vi "Certification Authority.vi"() -> ()   [LabVIEW 2013, in "Certification Authority.lvclass"]
uses:
  Certification Authority.lvclass
  certificate -- cluster.ctl
  certificate signature request (CA) -- cluster.ctl
  encryption key -- cluster.ctl
  initca -- cluster.ctl
  certificate signature request (Server) -- cluster.ctl
  <vilib>/Platform/browser.llb/Open URL in Default Browser (string).vi
  <vilib>/Platform/browser.llb/Open URL in Default Browser (path).vi
  <userlib>/_OpenG.lib/file/file.llb/Build Path - Traditional__ogtk.vi
  <userlib>/_OpenG.lib/file/file.llb/File Exists - Scalar__ogtk.vi
  <userlib>/_OpenG.lib/file/file.llb/Convert File Extension (String)__ogtk.vi
panel:
  in  "Tab Control":T1(tab)
  in  "Root Certificate":path
  in  "Root Private Key":path
  in  "Open Certificates Folder":bool
  in  "Open GitHub Project Page":bool
  in  "Hosts":string[](array[string])=["lvtls-ca.example", "www.lvtls-ca.example"]
  in  "Common Name":string="lvtls-ca.example"
  in  "Generate Root Certificate":bool
  out "CFSSL App found":bool
  out "Root Certificate found":bool
  in  "Generate Server Certificates":bool
  in  "Servers":cluster{"hosts":string[], "name":string}[](array[cluster])
  out "Certificates":T2(array[cluster])
  in  "Certificates and Keys":i32(listbox)
  out "Selected Certificate":string
  # "ROOT (CERTIFICATE AUTHORITY)\nIf you have a root certificate and private key, import it to generate server certificate files.\nIf you don't have a root certificate, fill in the fields in section 2 and generate one."
  # "GENERATE ROOT CERTIFICATE\nIf you don't have a root certificate, fill in the fields below and generate one."
  # "3- SERVERS\nList each server you want to create certificates for."
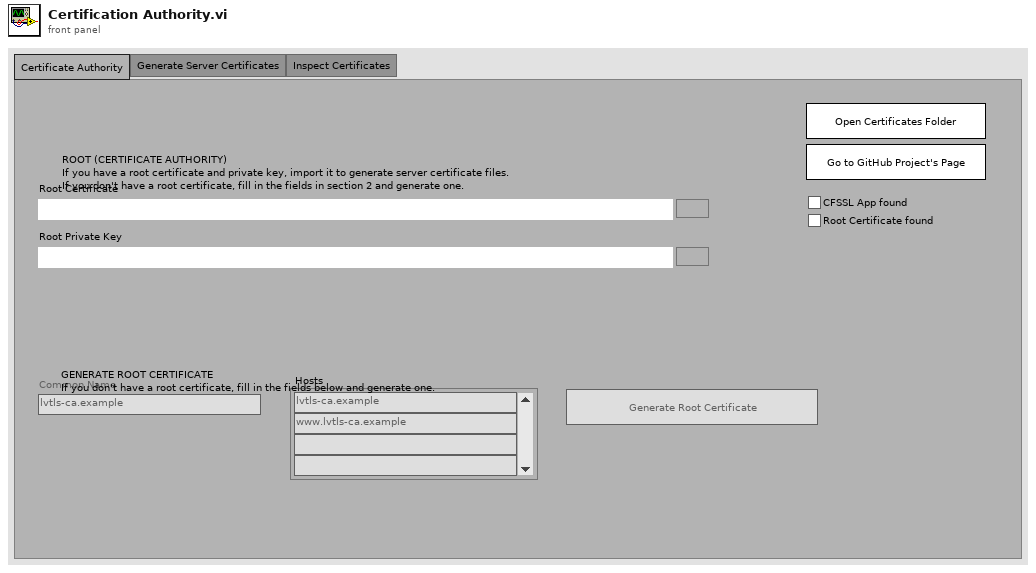
[diagram p1: front panel]
types:
  T1 = enum32{"Certificate Authority", "Generate Server Certificates", "Inspect Certificates"}
  T2 = cluster{"Type":string, "Decoded Certificate":string}[]
  T3 = enum32{"Invalid", "Standard", "Closed", "Hidden", "Minimized", "Maximized"}
  T4 = enum32{"invalid app kind", "Development System", "Run Time System", "Student Edition", "Embedded LabVIEW", "Evaluation", "Custom"}
  T5 = enum16{"open", "replace", "create", "open or create", "replace or create", "replace or create with confirmation"}
  T6 = typedef "Certification Authority.lvclass/certificate signature request (CA) -- cluster.ctl" = cluster{"CN":string, "hosts":string[], "key":T7, "ca":T8}
  T7 = typedef "Certification Authority.lvclass/encryption key -- cluster.ctl" = cluster{"algo":string, "size":u32}
  T8 = typedef "Certification Authority.lvclass/initca -- cluster.ctl" = cluster{"pathlen":u8, "expiry":string}
  T9 = typedef "Certification Authority.lvclass/certificate signature request (Server) -- cluster.ctl" = cluster{"CN":string, "hosts":string[], "key":T7}
  T10 = typedef "Certification Authority.lvclass/certificate -- cluster.ctl" = cluster{"cert":string, "csr":string, "key":string}
  T11 = cluster{"Core":cluster{"Current VI Reference":refnum<vi>, "Close Panel on Exit?":bool}, "CA":T10, "Server":T10, "cfssl path":path, "temp folder":path, "Certificates Folder":path, "Root name":string, "Root Certificate":path, "Root Private Key":path, "Active CN":string, "Active Hosts":string[], "next":i32, "Processing Queue":cluster{"hosts":string[], "name":string}[]}
  T12 = cluster{"Current VI Reference":refnum<vi>, "Close Panel on Exit?":bool}
  T13 = cluster{"Type":string, "Decoded String":string}[]
  T14 = enum8{"Enabled", "Disabled", "Disabled and Grayed Out"}
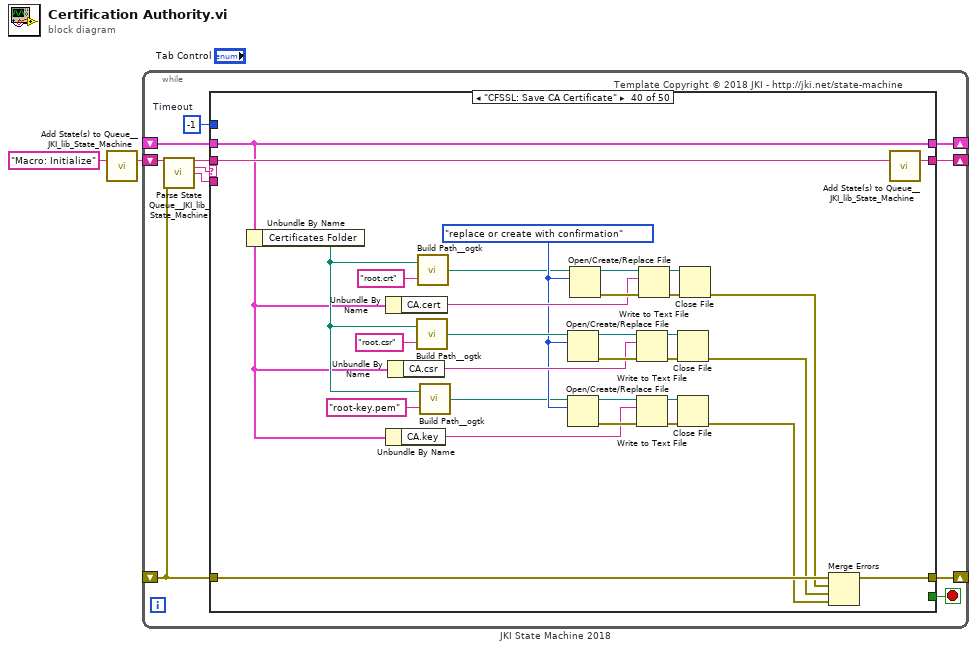
[diagram p0: block diagram]
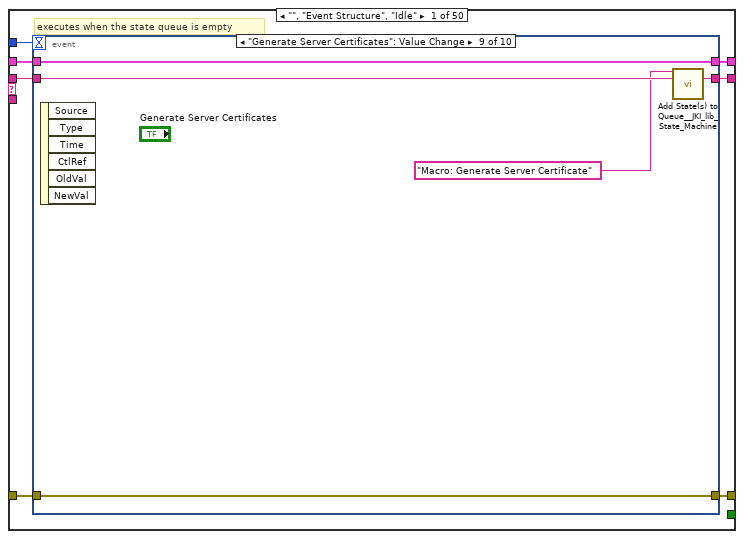
[diagram p2: hidden frame]
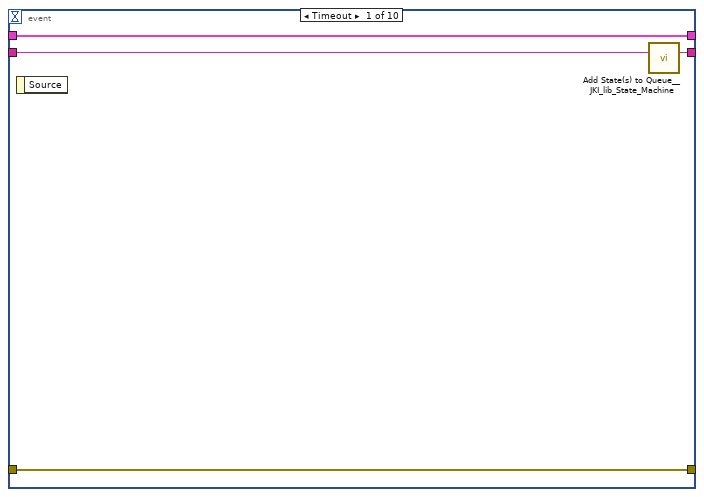
[diagram p3: hidden frame]
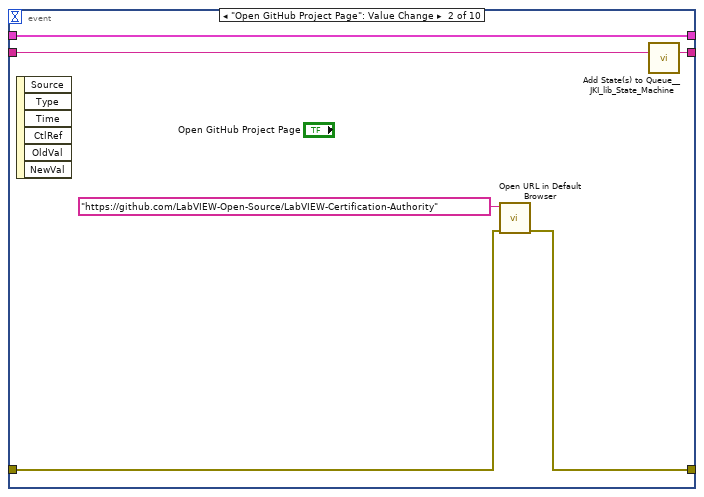
[diagram p4: hidden frame]
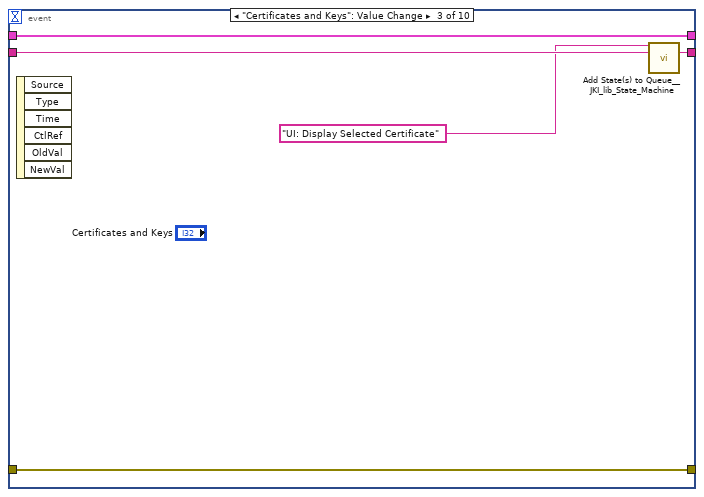
[diagram p5: hidden frame]
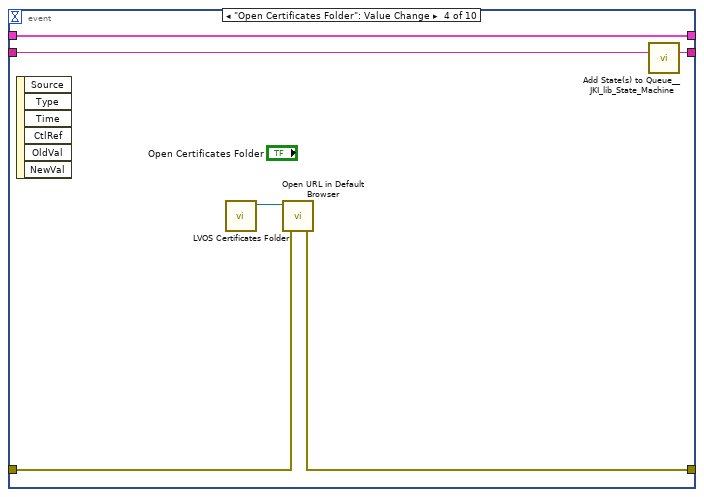
[diagram p6: hidden frame]
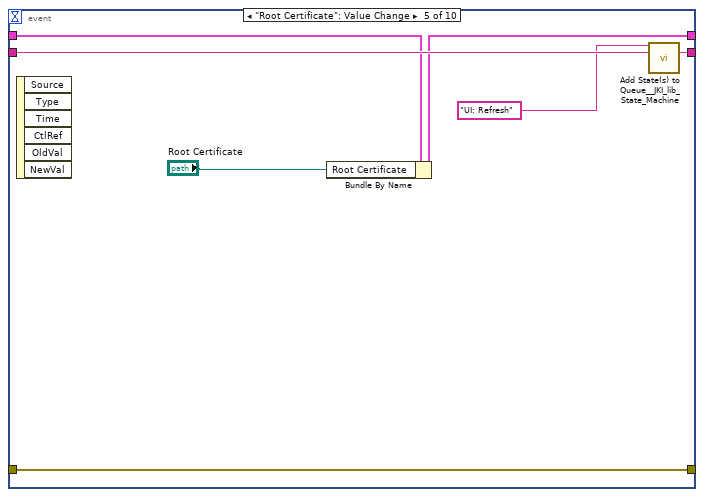
[diagram p7: hidden frame]
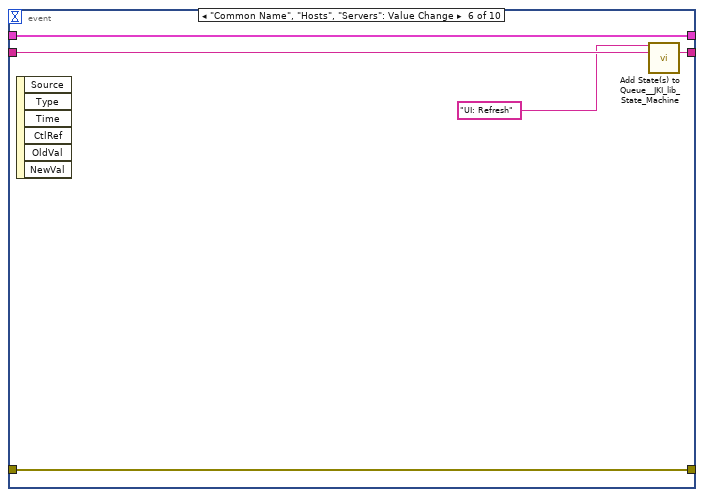
[diagram p8: hidden frame]
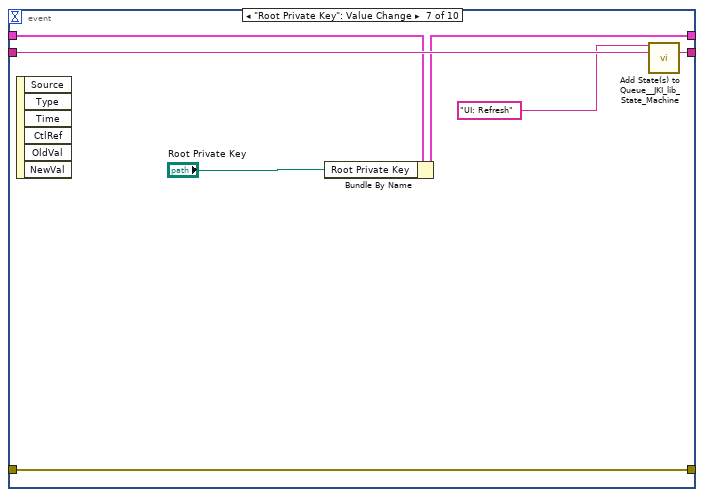
[diagram p9: hidden frame]
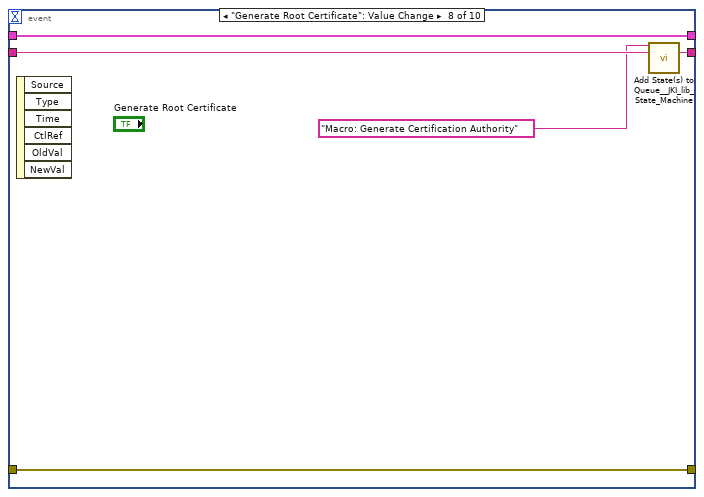
[diagram p10: hidden frame]
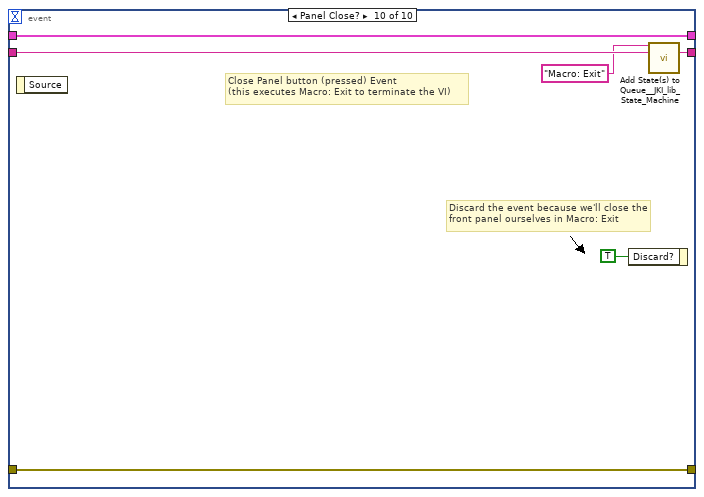
[diagram p11: hidden frame]
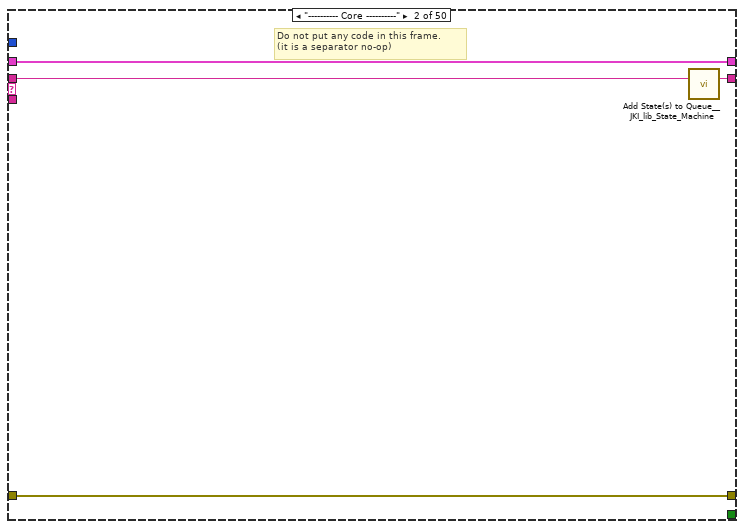
[diagram p12: hidden frame]
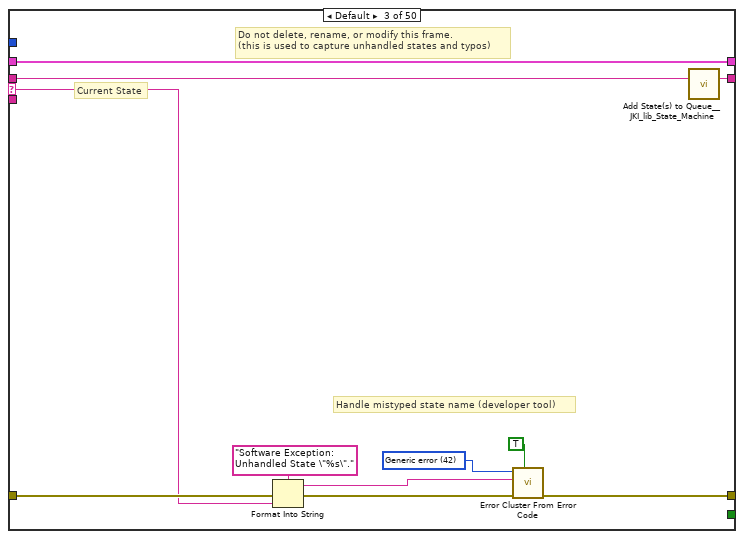
[diagram p13: hidden frame]
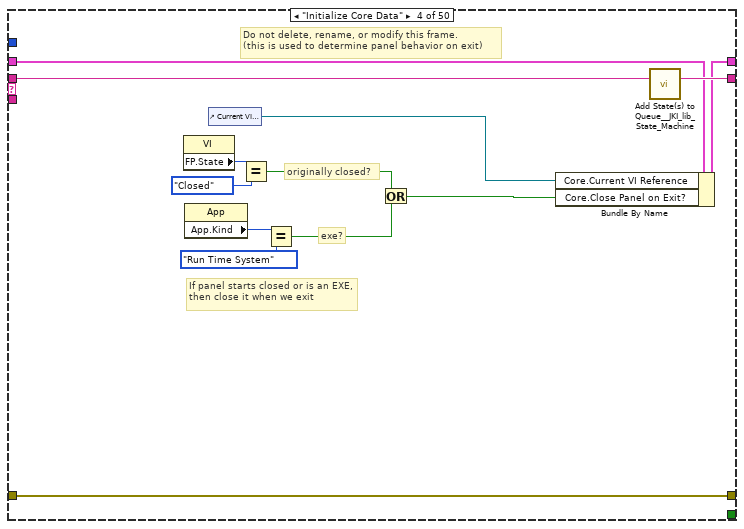
[diagram p14: hidden frame]
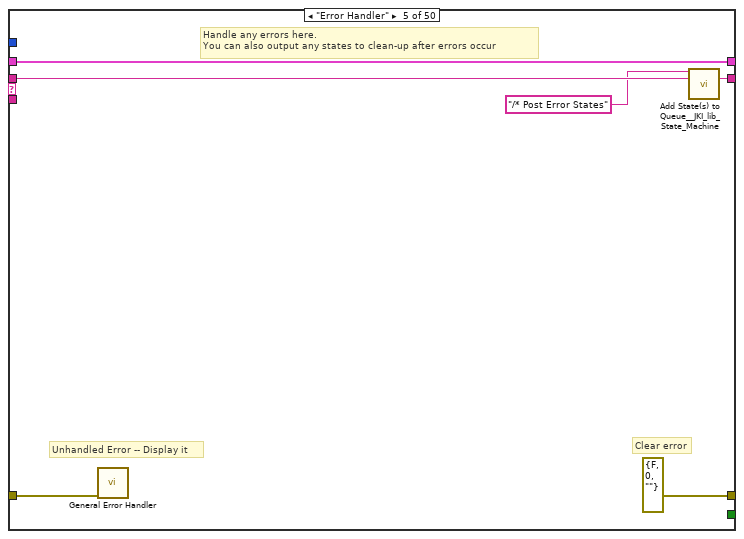
[diagram p15: hidden frame]
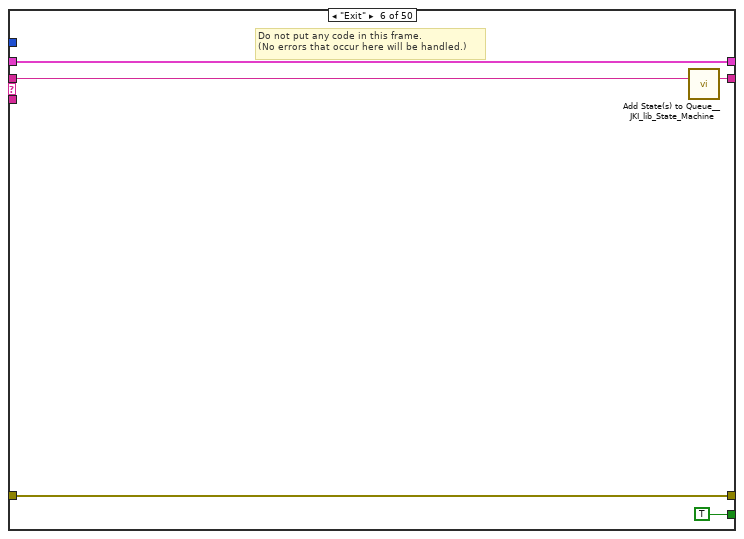
[diagram p16: hidden frame]
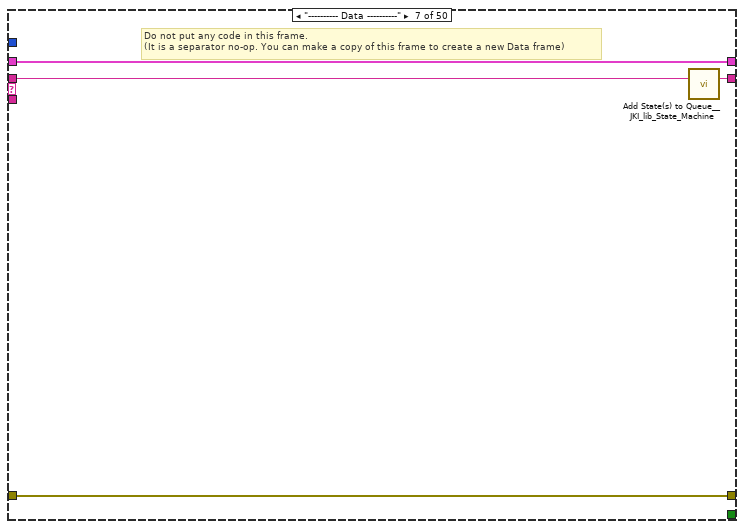
[diagram p17: hidden frame]
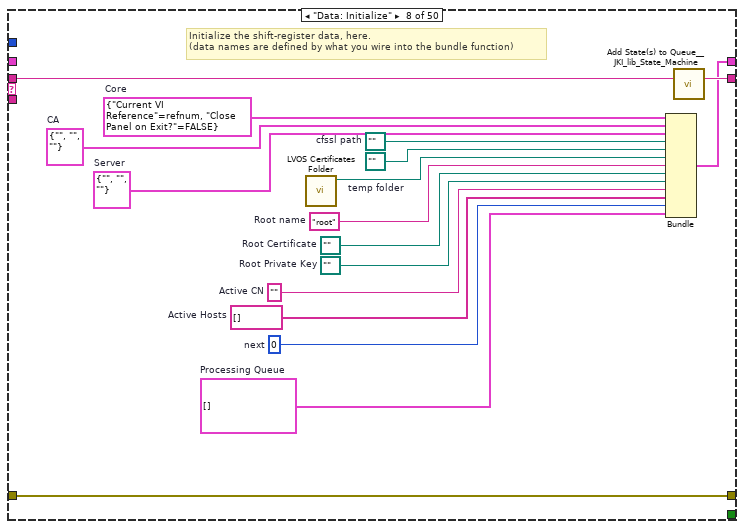
[diagram p18: hidden frame]
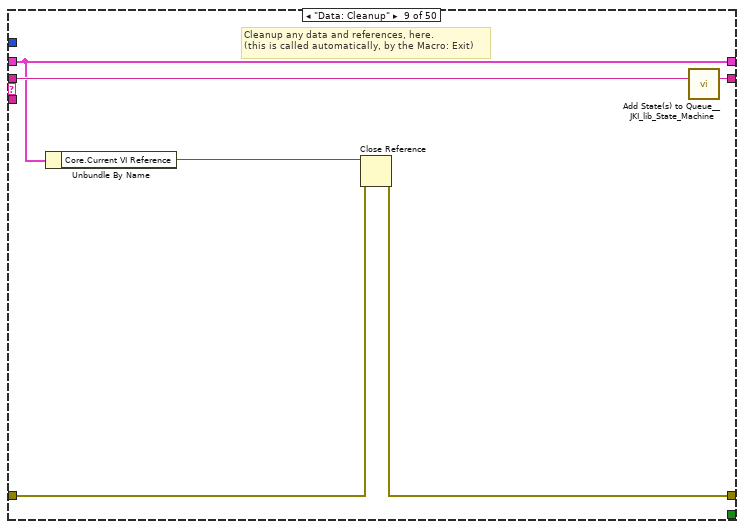
[diagram p19: hidden frame]
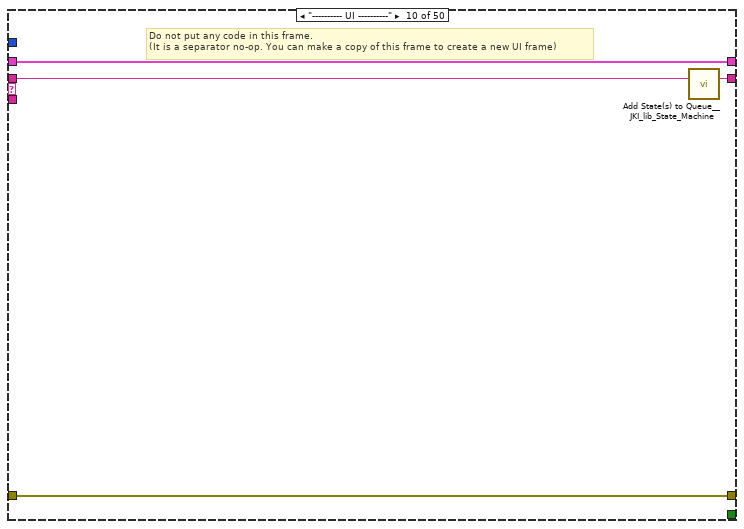
[diagram p20: hidden frame]
diagram:
  n1 = call <vilib>:"Add State(s) to Queue__JKI_lib_State_Machine.vi"("State(s) in (\"\")"="Macro: Initialize") -> ("States Out"=w2:string)  [unwired: 14 in]
  n2 = while "JKI State Machine 2018" {
    shift-right: [w6] -> _
    shift-left: _ -> [w5]
    shift-right: [w9] -> _
    shift-left: _ -> [w3]
    shift-right: [w8] -> _
    shift-left: w2 -> [w10]
    stop <- w7 stop-if-true
    w4 = -1  # Timeout
    # "Template Copyright © 2018 JKI - http://jki.net/state-machine"
    n3 = call <vilib>:"Parse State Queue__JKI_lib_State_Machine.vi"("State Queue"=w10, "Error In (no error)"=w3) -> ("Remaining States"=w12:string, "Current State"=w13:string, "Arguments"=w11:string)  [unwired: 11 in]
    n4 = case shown="\"CFSSL: Save CA Certificate\"" w13 {
      selector: w13 -> [_ _ w81 _ _ _ _ _ _ _ _ _ _ _ _ _ _ _ _ _ _ _ _ _ _ _ _ _ _ _ _ _ _ _ _ _ _ _ _ _ _ _ _ _ _ _ _ _ _ _]
      tunnel: w12 -> [w20 w80 w85 w104 w110 w115 w119 w136 w142 w146 w155 w166 w175 w230 w234 w238 w243 w249 w260 w329 w334 w339 w347 w352 w361 w366 w377 w381 w392 w405 w415 w442 w457 w472 w495 w516 w533 w543 w557 w588 w611 w637 w660 w692 w709 w726 w743 w760 w777 w794]
      tunnel: w11 -> [_ _ _ _ _ _ _ _ _ _ _ _ _ _ _ _ _ w244 w254 _ _ _ _ _ _ _ _ _ _ _ _ _ _ _ _ _ _ _ _ _ _ _ _ _ _ _ _ _ _ _]
      tunnel: w5 -> [w18 w77 w83 w97 w107 w113 w116 _ w137 w143 w153 w164 w173 w200 w231 w235 w240 w247 w256 w326 w331 w336 w343 w349 w358 w363 w374 w378 w389 w403 w413 w438 w446 w462 w493 w514 w526 w538 w555 w558 w604 w633 w650 w675 w701 w718 w735 w752 w769 w786]
      tunnel: [w17 w78 w87 w101 errorcluster {"status"=FALSE, "code"=0, "source"=""} ("error out") w112 w117 w133 w138 w144 w149 w161 w170 w228 w232 w236 w241 w245 w257 w327 w332 w337 w345 w350 w359 w364 w375 w379 w390 w398 w409 w440 w443 w459 w473 w502 w519 w534 w546 w561 w606 w634 w639 w676 w696 w713 w730 w747 w764 w781] -> w9
      tunnel: w3 -> [w16 w78 w86 w101 w106 w112 w117 w133 w139 w144 w150 w162 w170 w228 w232 w236 w241 w246 w258 w327 w332 w337 w345 w350 w359 w364 w375 w379 w390 w399 w408 w440 w444 w460 w474 w503 w520 w534 w544 w565 w607 w635 w642 w679 w698 w715 w732 w749 w766 w783]
      tunnel: [w19 w79 w84 w103 w109 w114 w118 w135 w141 w145 w154 w165 w174 w229 w233 w237 w242 w248 w259 w328 w333 w338 w346 w351 w360 w365 w376 w380 w391 w404 w414 w441 w456 w471 w494 w515 w532 w542 w556 w587 w610 w636 w659 w691 w708 w725 w742 w759 w776 w793] -> w8
      tunnel: [_ _ _ _ _ TRUE _ _ _ _ _ _ _ _ _ _ _ _ _ _ _ _ _ _ _ _ _ _ _ _ _ _ _ _ _ _ _ _ _ _ _ _ _ _ _ _ _ _ _ _] -> w7
      tunnel: [w15 w77 w83 w102 w107 w113 w116 w134 w137 w143 w153 w164 w173 w200 w231 w235 w240 w247 w256 w326 w331 w336 w342 w349 w358 w363 w374 w378 w388 w402 w413 w439 w447 w463 w493 w514 w526 w541 w555 w558 w603 w632 w650 w675 w701 w718 w735 w752 w769 w786] -> w6
      tunnel: w4 -> [w14 _ _ _ _ _ _ _ _ _ _ _ _ _ _ _ _ _ _ _ _ _ _ _ _ _ _ _ _ _ _ _ _ _ _ _ _ _ _ _ _ _ _ _ _ _ _ _ _ _]
      frame "", "Event Structure", "Idle" {
        # "executes when the state queue is empty"
        n5 = event shown="[8] \"Generate Server Certificates\": Value Change" {
          selector: _ -> [_ _ _ _ _ _ _ _ _ _]
          dyn-events: _ -> [_ _ _ _ _ _ _ _ _ _]
          timeout: w14 -> [_ _ _ _ _ _ _ _ _ _]
          tunnel: w20 -> [w24 w30 w35 w41 w48 w53 w60 w65 w70 w76]
          tunnel: [w23 w29 w34 w40 w47 w52 w59 w64 w69 w75] -> w19
          tunnel: w18 -> [w21 w28 w32 w39 w45 w49 w57 w62 w67 w73]
          tunnel: [w22 w25 w33 w36 w46 w51 w58 w63 w68 w74] -> w17
          tunnel: w16 -> [w22 w26 w33 w37 w46 w51 w58 w63 w68 w74]
          tunnel: [w21 w28 w32 w39 w44 w49 w56 w62 w67 w73] -> w15
          event Timeout {
            n6 = event-data() -> ()  [unwired: 1 in, 1 out]
            n7 = call <vilib>:"Add State(s) to Queue__JKI_lib_State_Machine.vi"("State(s) in (\"\")"=w24) -> ("States Out"=w23:string)  [unwired: 14 in]
          }
          event "Open GitHub Project Page": Value Change {
            n8 = event-data() -> ()  [unwired: 1 in, 6 out]
            n9 = call-poly <vilib>:"Open URL in Default Browser.vi"("error in (no error)"=w26, "URL"="https://github.com/LabVIEW-Open-Source/LabVIEW-Certification-Authority") -> ("error out"=w25:errorcluster)  [unwired: 4 in, 1 out]
            n10 = call <vilib>:"Add State(s) to Queue__JKI_lib_State_Machine.vi"("State(s) in (\"\")"=w30) -> ("States Out"=w29:string)  [unwired: 14 in]
          }
          event "Certificates and Keys": Value Change {
            n11 = event-data() -> ()  [unwired: 1 in, 6 out]
            n12 = call <vilib>:"Add State(s) to Queue__JKI_lib_State_Machine.vi"("State(s) in Front (\"\")"="UI: Display Selected Certificate", "State(s) in (\"\")"=w35) -> ("States Out"=w34:string)  [unwired: 13 in]
          }
          event "Open Certificates Folder": Value Change {
            n13 = event-data() -> ()  [unwired: 1 in, 6 out]
            n14 = call "LVOS Certificates Folder.vi"() -> ("Certificates Folder"=w38:path)  [unwired: 10 in, 1 out]
            n15 = call-poly <vilib>:"Open URL in Default Browser.vi"("error in (no error)"=w37, "path"=w38) -> ("error out"=w36:errorcluster)  [unwired: 4 in, 1 out]
            n16 = call <vilib>:"Add State(s) to Queue__JKI_lib_State_Machine.vi"("State(s) in (\"\")"=w41) -> ("States Out"=w40:string)  [unwired: 14 in]
          }
          event "Root Certificate": Value Change {
            n17 = event-data() -> ()  [unwired: 1 in, 6 out]
            n18 = Bundle By Name(cluster=w45, "Root Certificate"="Root Certificate") -> (w44:T11)
            n19 = call <vilib>:"Add State(s) to Queue__JKI_lib_State_Machine.vi"("State(s) in Front (\"\")"="UI: Refresh", "State(s) in (\"\")"=w48) -> ("States Out"=w47:string)  [unwired: 13 in]
          }
          event "Common Name", "Hosts", "Servers": Value Change {
            n20 = event-data() -> ()  [unwired: 1 in, 6 out]
            n21 = call <vilib>:"Add State(s) to Queue__JKI_lib_State_Machine.vi"("State(s) in Front (\"\")"="UI: Refresh", "State(s) in (\"\")"=w53) -> ("States Out"=w52:string)  [unwired: 13 in]
          }
          event "Root Private Key": Value Change {
            n22 = event-data() -> ()  [unwired: 1 in, 6 out]
            n23 = Bundle By Name(cluster=w57, "Root Private Key"="Root Private Key") -> (w56:T11)
            n24 = call <vilib>:"Add State(s) to Queue__JKI_lib_State_Machine.vi"("State(s) in Front (\"\")"="UI: Refresh", "State(s) in (\"\")"=w60) -> ("States Out"=w59:string)  [unwired: 13 in]
          }
          event "Generate Root Certificate": Value Change {
            n25 = event-data() -> ()  [unwired: 1 in, 6 out]
            n26 = call <vilib>:"Add State(s) to Queue__JKI_lib_State_Machine.vi"("State(s) in Front (\"\")"="Macro: Generate Certification Authority", "State(s) in (\"\")"=w65) -> ("States Out"=w64:string)  [unwired: 13 in]
          }
          event "Generate Server Certificates": Value Change {
            n27 = event-data() -> ()  [unwired: 1 in, 6 out]
            n28 = call <vilib>:"Add State(s) to Queue__JKI_lib_State_Machine.vi"("State(s) in Front (\"\")"="Macro: Generate Server Certificate", "State(s) in (\"\")"=w70) -> ("States Out"=w69:string)  [unwired: 13 in]
          }
          event Panel Close? {
            # "Discard the event because we'll close the front panel ourselves in Macro: Exit"
            # "Close Panel button (pressed) Event\n(this executes Macro: Exit to terminate the VI)"
            n29 = event-data() -> ()  [unwired: 1 in, 1 out]
            n30 = event-data("Discard?"=TRUE) -> ()  [unwired: 1 in, 1 out]
            n31 = call <vilib>:"Add State(s) to Queue__JKI_lib_State_Machine.vi"("State(s) in Front (\"\")"="Macro: Exit", "State(s) in (\"\")"=w76) -> ("States Out"=w75:string)  [unwired: 13 in]
          }
        }
      }
      frame "---------- Core ----------" {
        # "Do not put any code in this frame.\n(it is a separator no-op)"
        n32 = call <vilib>:"Add State(s) to Queue__JKI_lib_State_Machine.vi"("State(s) in (\"\")"=w80) -> ("States Out"=w79:string)  [unwired: 14 in]
      }
      frame Default {
        w90 = 42 items=["No error", "Argument error", "Memory is full", "Out of zone", "End of file", "File already open", "Generic file I/O error", "File not found", "File permission error", "Disk is full", "Duplicate path", "Too many files open", "System feature not enabled", "Resource file not found", "Cannot add resource", "Resource not found", "Image not found", "Image memory error", "Pen does not exist", "Config type invalid", "Config token not found", "Config parse error", "Config memory error", "Bad external code format", "Bad external code offset", "External code not present", "Null window", "Destroy window error", "Null menu", "Print aborted", "Bad print record", "Print driver error", "Windows error during printing", "Memory error during printing", "Print dialog error", "Generic print error", "Invalid device refnum", "Device not found", "Device parameter error", "Device unit error", "Cannot open device", "Device call aborted", "Generic error", "Cancelled by user", "Object ID too low", "Object ID too high", "Object not in heap", "Unknown heap", "Unknown object (invalid DefProc)", "Unknown object (DefProc not in table)", "Message out of range", "Invalid (null) method", "Unknown message", "Manager call not supported", "Bad address", "Network operation in progress", "Network operation timed out", "Connection is busy", "Network attribute not supported", "Network error", "Address in use", "System out of memory", "Connection aborted", "Connection refused", "Not connected", "Already connected", "Connection closed", "Initialization error (interapplication manager)", "Bad occurrence", "Wait on unbound occurrence handler", "Occurrence queue overflow", "Datalog type conflict", "Unused", "Unrecognized type (interapplication manager)", "Memory corrupt", "Failed to make temporary DLL", "Old CIN version", "Drag socket not found", "Failed to load drop-object", "Failed to register OLE object", "Failed to release OLE object", "Format specifier type mismatch", "Unknown format specifier", "Too few format specifiers", "Too many format specifiers", "Scan failed", "Newer CIN version", "Error converting to variant", "Runtime menu error", "Password tampered", "Variant attribute not found", "Incompatible variant data type", "Event data is not available", "Event Store is not present", "Occurrence is not found", "Event Queue is not created", "Event info is not available", "Refnum passed is NULL", "Error retrieving Class GUID", "Error retrieving CoClass GUID", "Error retrieving TypeLib GUID.", "Bad built application magic bytes.", "Specific driver is different from the specific driver associated with the Logical Name.", "There is no session opened to the class driver.", "Max Error", "MAX - Error with config objects", "MAX - Error loading configuration", "MAX - Group not supported"]
        # "Current State"
        # "Do not delete, rename, or modify this frame.\n(this is used to capture unhandled states and typos)"
        # "Handle mistyped state name (developer tool)"
        n33 = Format Into String(format string="Software Exception: Unhandled State \"%s\"." ("message"), error in=w86, w81) -> (resulting string=w89:string, error out=w88:errorcluster)  [unwired: 1 in]
        n34 = call <vilib>:"Error Cluster From Error Code.vi"("show call chain? (False)"=TRUE, "error in (no error)"=w88, "error message (\"\")"=w89, "error code (0)"=w90) -> ("error out"=w87:errorcluster)  [unwired: 5 in]
        n35 = call <vilib>:"Add State(s) to Queue__JKI_lib_State_Machine.vi"("State(s) in (\"\")"=w85) -> ("States Out"=w84:string)  [unwired: 14 in]
      }
      frame "Initialize Core Data" {
        # "Do not delete, rename, or modify this frame.\n(this is used to determine panel behavior on exit)"
        # "originally closed?"
        # "exe?"
        # "If panel starts closed or is an EXE, then close it when we exit"
        n36 = property class="VI"() -> ("FP.State"=w94:T3)  [unwired: 2 in, 2 out]
        n37 = property class="App"() -> ("App.Kind"=w100:T4)  [unwired: 2 in, 2 out]
        n38 = control-ref of="Current VI Reference"() -> (w95:refnum<vi>)
        n39 = Equal?(x=w94, y=T3."Closed" ("Front Panel Window:State")) -> (x = y?=w92:bool)
        n40 = Equal?(x=w100, y=T4."Run Time System" ("Application:Kind")) -> (x = y?=w98:bool)
        n41 = Or(x=w92, y=w98) -> (x .or. y?=w96:bool)
        n42 = Bundle By Name(cluster=w97, "Core.Current VI Reference"=w95, "Core.Close Panel on Exit?"=w96) -> (w102:T11)
        n43 = call <vilib>:"Add State(s) to Queue__JKI_lib_State_Machine.vi"("State(s) in (\"\")"=w104) -> ("States Out"=w103:string)  [unwired: 14 in]
      }
      frame "Error Handler" {
        # "Unhandled Error -- Display it"
        # "Handle any errors here.\nYou can also output any states to clean-up after errors occur"
        # "Clear error"
        n44 = call <vilib>:"General Error Handler.vi"("error in (no error)"=w106) -> ()  [unwired: 10 in, 5 out]
        n45 = call <vilib>:"Add State(s) to Queue__JKI_lib_State_Machine.vi"("State(s) in Front (\"\")"="/* Post Error States", "State(s) in (\"\")"=w110) -> ("States Out"=w109:string)  [unwired: 13 in]
      }
      frame "Exit" {
        # "Do not put any code in this frame.\n(No errors that occur here will be handled.)"
        n46 = call <vilib>:"Add State(s) to Queue__JKI_lib_State_Machine.vi"("State(s) in (\"\")"=w115) -> ("States Out"=w114:string)  [unwired: 14 in]
      }
      frame "---------- Data ----------" {
        # "Do not put any code in this frame.\n(It is a separator no-op. You can make a copy of this frame to create a new Data frame)"
        n47 = call <vilib>:"Add State(s) to Queue__JKI_lib_State_Machine.vi"("State(s) in (\"\")"=w119) -> ("States Out"=w118:string)  [unwired: 14 in]
      }
      frame "Data: Initialize" {
        w120 = cluster{"hosts":string[], "name":string}[] []  # Processing Queue
        w121 = 0  # next
        w123 = string[] []  # Active Hosts
        w124 = ""  # Active CN
        w125 = path ""  # Root Private Key
        w126 = path ""  # Root Certificate
        w127 = "root"  # Root name
        w128 = path ""  # temp folder
        w129 = path ""  # cfssl path
        w130 = T10 {"cert"="", "csr"="", "key"=""}  # Server
        w131 = T10 {"cert"="", "csr"="", "key"=""}  # CA
        w132 = T12 {"Current VI Reference"=refnum, "Close Panel on Exit?"=FALSE}  # Core
        # "Initialize the shift-register data, here.\n(data names are defined by what you wire into the bundle function)"
        n48 = call "LVOS Certificates Folder.vi"() -> ("Certificates Folder"=w122:path)  [unwired: 10 in, 1 out]
        n49 = Bundle("Core"=w132, "CA"=w131, "Server"=w130, "cfssl path"=w129, "temp folder"=w128, "Certificates Folder"=w122, "Root name"=w127, "Root Certificate"=w126, "Root Private Key"=w125, "Active CN"=w124, "Active Hosts"=w123, "next"=w121, "Processing Queue"=w120) -> (w134:T11)  [unwired: 1 in]
        n50 = call <vilib>:"Add State(s) to Queue__JKI_lib_State_Machine.vi"("State(s) in (\"\")"=w136) -> ("States Out"=w135:string)  [unwired: 14 in]
      }
      frame "Data: Cleanup" {
        # "Cleanup any data and references, here.\n(this is called automatically, by the Macro: Exit)"
        n51 = Unbundle By Name(w137) -> ("Core.Current VI Reference"=w140:refnum<vi>)
        n52 = Close Reference(reference=w140, error in (no error)=w139) -> (error out=w138:errorcluster)
        n53 = call <vilib>:"Add State(s) to Queue__JKI_lib_State_Machine.vi"("State(s) in (\"\")"=w142) -> ("States Out"=w141:string)  [unwired: 14 in]
      }
      frame "---------- UI ----------" {
        # "Do not put any code in this frame.\n(It is a separator no-op. You can make a copy of this frame to create a new UI frame)"
        n54 = call <vilib>:"Add State(s) to Queue__JKI_lib_State_Machine.vi"("State(s) in (\"\")"=w146) -> ("States Out"=w145:string)  [unwired: 14 in]
      }
      frame "UI: Initialize" {
        # "Initialize the User Interface, here.\n(this is called automatically, by the Macro: Init)"
        n55 = property on="Certificates and Keys" class="LstBox (strict)"("Item Names"=string[] []) -> ()  [unwired: 2 in, 2 out]
        n56 = local write "Tab Control"(0) -> ()
        n57 = call "LVOS Certificates Folder.vi"() -> ("Certificates Folder"=w152:path)  [unwired: 10 in, 1 out]
        n58 = call <userlib>:"Create Dir if Non-Existant__ogtk.vi"("error in (no error)"=w150, "Directory Path"=w152) -> ("error out"=w149:errorcluster, "dup Directory Path"=w151:path)  [unwired: 7 in, 1 out]
        n59 = invoke on="Servers" class="Arr (strict)" method="Reinit To Default"() -> ()  [unwired: 3 in, 3 out]
        n60 = property on="Root Private Key" class="Path"("StartPath"=w151) -> ()  [unwired: 2 in, 2 out]
        n61 = property on="Root Certificate" class="Path"("StartPath"=w151) -> ()  [unwired: 2 in, 2 out]
        n62 = call <vilib>:"Add State(s) to Queue__JKI_lib_State_Machine.vi"("State(s) in (\"\")"=w155) -> ("States Out"=w154:string)  [unwired: 14 in]
      }
      frame "UI: List Certificates" {
        n63 = call "LVOS Certificates Folder.vi"() -> ("Certificates Folder"=w163:path)  [unwired: 10 in, 1 out]
        n64 = call <userlib>:"Create Dir if Non-Existant__ogtk.vi"("error in (no error)"=w162, "Directory Path"=w163) -> ("error out"=w161:errorcluster, "dup Directory Path"=w160:path)  [unwired: 7 in, 1 out]
        n65 = call <userlib>:"List Directory__ogtk.vi"("pattern"="*.pem; *.crt; *.csr", "directory path"=w160) -> ("file names"=w158:string[])  [unwired: 2 in, 3 out]
        n66 = Sort 1D Array(array=w158) -> (sorted array=w157:string[])
        n67 = property on="Certificates and Keys" class="LstBox (strict)"("Item Names"=w157, "Value"=-1 ("Trusted Certificates")) -> ()  [unwired: 2 in, 2 out]
        n68 = call <vilib>:"Add State(s) to Queue__JKI_lib_State_Machine.vi"("State(s) in (\"\")"=w166) -> ("States Out"=w165:string)  [unwired: 14 in]
      }
      frame "UI: Display Selected Certificate" {
        n69 = property on="Certificates and Keys" class="LstBox (strict)"() -> ("Item Names"=w172:string[], "Value"=w171:i32)  [unwired: 2 in, 2 out]
        n70 = Index Array(array=w172, index=w171) -> (element=w169:string)
        n71 = case shown="Default" w169 {
          selector: w169 -> [w182 _]
          tunnel: [w176 _] -> w168
          frame Default {
            n72 = call "LVOS Certificates Folder.vi"() -> ("Certificates Folder"=w183:path)  [unwired: 10 in, 1 out]
            n73 = call-poly <userlib>:"Build Path__ogtk.vi"("name or relative path"=w182, "base path"=w183) -> ("appended path"=w178:path)
            n74 = call-poly <userlib>:"File Exists__ogtk.vi"("file path"=w178) -> ("is directory"=w181:bool, "exists"=w180:bool)  [unwired: 6 in]
            n75 = Empty String/Path?(string/path=w178) -> (empty?=w179:bool)
            n76 = Compound Arithmetic op=AND(invert w181, w180, invert w179) -> (w177:bool)
            n77 = case shown="True" w177 {
              tunnel: w178 -> [_ w185]
              tunnel: [_ w184] -> w176
              frame False {
              }
              frame True {
                n78 = Open/Create/Replace File(file path (use dialog)=w185, operation (0:open)=T5."open", access (0:read/write)=enum16{"read/write", "read-only", "write-only"}."read-only") -> (refnum out=w190:refnum<file>, error out=w191:errorcluster)  [unwired: 3 in, 1 out]
                n79 = Read from Text File(file (use dialog)=w190, error in=w191) -> (refnum out=w188:refnum<file>, text=w184:string, error out=w189:errorcluster)  [unwired: 2 in, 1 out]
                n80 = Close File(refnum=w188, error in=w189) -> ()  [unwired: 2 out]
              }
            }
          }
          frame "" {
          }
        }
        "Selected Certificate" <- w168
        n81 = call "Inspect Certificate.vi"("Certificate string"=w168) -> ("Certificates"=→"Certificates":T13)  [unwired: 10 in]
        n82 = call <vilib>:"Add State(s) to Queue__JKI_lib_State_Machine.vi"("State(s) in (\"\")"=w175) -> ("States Out"=w174:string)  [unwired: 14 in]
      }
      frame "UI: Refresh" {
        w205 = T14."Disabled and Grayed Out" ("Disabled")
        w204 = T14."Enabled" ("Disabled")
        n83 = Unbundle By Name(w200) -> ("Certificates Folder"=w225:path)
        n84 = Unbundle By Name(w200) -> ("Root Certificate"=w202:path, "Root Private Key"=w201:path)
        n85 = local read "Common Name"() -> (w209:string)
        n86 = local read "Servers"() -> (w222:cluster{"hosts":string[], "name":string}[])
        n87 = Unbundle By Name(w200) -> ("cfssl path"=w199:path)
        n88 = local read "Hosts"() -> (w208:string[])
        n89 = Not A Number/Path/Refnum?(number/path/refnum=w199) -> (NaN/Path/Refnum?=w194:bool)
        n90 = local write "Root Private Key"(w201) -> ()
        n91 = call-poly <userlib>:"File Exists__ogtk.vi"("file path"=w225) -> ("is directory"=w223:bool, "exists"=w224:bool)  [unwired: 6 in]
        n92 = Empty String/Path?(string/path=w225) -> (empty?=w226:bool)
        n93 = Empty Array?(array=w222) -> (empty?=w227:bool)
        n94 = Empty String/Path?(string/path=w209) -> (empty?=w207:bool)
        n95 = local write "Root Certificate"(w202) -> ()
        n96 = call-poly <userlib>:"File Exists__ogtk.vi"("file path"=w202) -> ("is directory"=w219:bool, "exists"=w218:bool)  [unwired: 6 in]
        n97 = call-poly <userlib>:"File Exists__ogtk.vi"("file path"=w201) -> ("is directory"=w214:bool, "exists"=w215:bool)  [unwired: 6 in]
        n98 = Empty String/Path?(string/path=w202) -> (empty?=w217:bool)
        n99 = Empty String/Path?(string/path=w201) -> (empty?=w216:bool)
        n100 = Empty Array?(array=w208) -> (empty?=w206:bool)
        n101 = Compound Arithmetic op=AND(invert w219, w218, invert w217) -> (w213:bool)
        n102 = Compound Arithmetic op=AND(invert w214, w215, invert w216) -> (w212:bool)
        n103 = Compound Arithmetic op=AND(w213, w212) -> (w192:bool)
        "Root Certificate found" <- w192
        n104 = Not(x=w194) -> (.not. x?=→"CFSSL App found":bool)
        n105 = Not(x=w192) -> (.not. x?=w196:bool)
        n106 = Compound Arithmetic op=AND(w196, invert w194) -> (w197:bool)
        n107 = Compound Arithmetic op=AND(w192, w223, w224, invert w226, invert w227, invert w194) -> (w220:bool)
        n108 = Compound Arithmetic op=AND(w196, invert w194) -> (w195:bool)
        n109 = Compound Arithmetic op=AND(invert w207, invert w206, w196, invert w194) -> (w198:bool)
        n110 = Select(t=w204, s=w195, f=w205) -> (s? t:f=w210:T14)
        n111 = Select(t=w204, s=w197, f=w205) -> (s? t:f=w211:T14)
        n112 = Select(t=w204, s=w198, f=w205) -> (s? t:f=w203:T14)
        n113 = Select(t=w204, s=w220, f=w205) -> (s? t:f=w221:T14)
        n114 = property on="Generate Root Certificate" class="Bool"("DisabledEnum"=w203) -> ()  [unwired: 2 in, 2 out]
        n115 = property on="Generate Server Certificates" class="Bool"("DisabledEnum"=w221) -> ()  [unwired: 2 in, 2 out]
        n116 = property on="Common Name" class="Str"("DisabledEnum"=w210) -> ()  [unwired: 2 in, 2 out]
        n117 = property on="hostname" class="Str"("DisabledEnum"=w211) -> ()  [unwired: 2 in, 2 out]
        n118 = call <vilib>:"Add State(s) to Queue__JKI_lib_State_Machine.vi"("State(s) in (\"\")"=w230) -> ("States Out"=w229:string)  [unwired: 14 in]
      }
      frame "UI: Display CA" {
        n119 = Unbundle By Name(w231) -> ()  [unwired: 1 out]
        n120 = call <vilib>:"Add State(s) to Queue__JKI_lib_State_Machine.vi"("State(s) in (\"\")"=w234) -> ("States Out"=w233:string)  [unwired: 14 in]
      }
      frame "UI: Display Server Cert" {
        n121 = Unbundle By Name(w235) -> ()  [unwired: 1 out]
        n122 = call <vilib>:"Add State(s) to Queue__JKI_lib_State_Machine.vi"("State(s) in (\"\")"=w238) -> ("States Out"=w237:string)  [unwired: 14 in]
      }
      frame "UI: Show Temporary Folder" {
        n123 = Unbundle By Name(w240) -> ("temp folder"=w239:path)
        n124 = call-poly <vilib>:"Open URL in Default Browser.vi"("path"=w239) -> ()  [unwired: 5 in, 2 out]
        n125 = call <vilib>:"Add State(s) to Queue__JKI_lib_State_Machine.vi"("State(s) in (\"\")"=w243) -> ("States Out"=w242:string)  [unwired: 14 in]
      }
      frame "UI: Cursor Set" {
        # "Argument"
        # "Set and Unset Cursor Busy.\n(Usage: \"UI: Cursor Set >> Busy|Idle\")"
        n126 = case shown="\"Idle\", Default" w244 {
          tunnel: w246 -> [w251 w253]
          tunnel: [w250 w252] -> w245
          frame "Idle", Default {
            n127 = call <vilib>:"Unset Busy.vi"("error in (no error)"=w251) -> ("error out"=w250:errorcluster)  [unwired: 10 in]
          }
          frame "Busy" {
            n128 = call <vilib>:"Set Busy.vi"("error in (no error)"=w253) -> ("error out"=w252:errorcluster)  [unwired: 9 in, 1 out]
          }
        }
        n129 = call <vilib>:"Add State(s) to Queue__JKI_lib_State_Machine.vi"("State(s) in (\"\")"=w249) -> ("States Out"=w248:string)  [unwired: 14 in]
      }
      frame "UI: Front Panel State" {
        # "Argument"
        # "Set Front Panel Open or Closed\n(Usage: \"UI: Front Panel State >> Open|Close\")"
        n130 = Unbundle By Name(w256) -> ("Core.Current VI Reference"=w255:refnum<vi>)
        n131 = case shown="\"Minimize\", \"Minimized\"" w254 {
          tunnel: w258 -> [w266 w281 w292 w305 w318]
          tunnel: [w268 w282 w294 w307 w320] -> w257
          tunnel: w255 -> [w267 w279 w293 w306 w319]
          frame "Open", "Standard", Default {
            w261 = T3."Standard" ("State")
            n132 = property class="VI"(reference=w267, error in=w266) -> (reference out=w264:refnum<vi>, error out=w265:errorcluster, "FP.State"=w263:T3)
            n133 = Not Equal?(x=w263, y=w261) -> (x != y?=w262:bool)
            n134 = case shown="True" w262 {
              tunnel: [w272 w274] -> w268
              tunnel: w265 -> [w271 w274]
              tunnel: w264 -> [w270 _]
              tunnel: w261 -> [w269 _]
              frame True {
                n135 = invoke class="VI" method="FP.Open"(reference=w270, error in=w271, "Activate"=TRUE, "State"=w269) -> (error out=w272:errorcluster)  [unwired: 1 in, 4 out]
              }
              frame False {
              }
            }
          }
          frame "Close", "Closed" {
            n136 = property class="VI"(reference=w279, error in=w281) -> (reference out=w278:refnum<vi>, error out=w280:errorcluster, "FP.State"=w276:T3)
            n137 = Not Equal?(x=w276, y=T3."Closed" ("Front Panel Window:State")) -> (x != y?=w275:bool)
            n138 = case shown="True" w275 {
              tunnel: [w283 w286] -> w282
              tunnel: w280 -> [w283 w285]
              tunnel: w278 -> [_ w284]
              frame False {
              }
              frame True {
                n139 = invoke class="VI" method="FP.Close"(reference=w284, error in=w285) -> (error out=w286:errorcluster)  [unwired: 1 in, 2 out]
              }
            }
          }
          frame "Hidden", "Hide" {
            w287 = T3."Hidden" ("State")
            n140 = property class="VI"(reference=w293, error in=w292) -> (reference out=w290:refnum<vi>, error out=w291:errorcluster, "FP.State"=w289:T3)
            n141 = Not Equal?(x=w289, y=w287) -> (x != y?=w288:bool)
            n142 = case shown="True" w288 {
              tunnel: [w298 w299] -> w294
              tunnel: w291 -> [w297 w299]
              tunnel: w290 -> [w296 _]
              tunnel: w287 -> [w295 _]
              frame True {
                n143 = invoke class="VI" method="FP.Open"(reference=w296, error in=w297, "State"=w295) -> (error out=w298:errorcluster)  [unwired: 2 in, 4 out]
              }
              frame False {
              }
            }
          }
          frame "Minimize", "Minimized" {
            w300 = T3."Minimized" ("State")
            n144 = property class="VI"(reference=w306, error in=w305) -> (reference out=w303:refnum<vi>, error out=w304:errorcluster, "FP.State"=w302:T3)
            n145 = Not Equal?(x=w302, y=w300) -> (x != y?=w301:bool)
            n146 = case shown="True" w301 {
              tunnel: [w311 w312] -> w307
              tunnel: w304 -> [w310 w312]
              tunnel: w303 -> [w309 _]
              tunnel: w300 -> [w308 _]
              frame True {
                n147 = invoke class="VI" method="FP.Open"(reference=w309, error in=w310, "State"=w308) -> (error out=w311:errorcluster)  [unwired: 2 in, 4 out]
              }
              frame False {
              }
            }
          }
          frame "Maximize", "Maximized" {
            w313 = T3."Maximized" ("State")
            n148 = property class="VI"(reference=w319, error in=w318) -> (reference out=w316:refnum<vi>, error out=w317:errorcluster, "FP.State"=w315:T3)
            n149 = Not Equal?(x=w315, y=w313) -> (x != y?=w314:bool)
            n150 = case shown="True" w314 {
              tunnel: [w324 w325] -> w320
              tunnel: w317 -> [w323 w325]
              tunnel: w316 -> [w322 _]
              tunnel: w313 -> [w321 _]
              frame True {
                n151 = invoke class="VI" method="FP.Open"(reference=w322, error in=w323, "State"=w321) -> (error out=w324:errorcluster)  [unwired: 2 in, 4 out]
              }
              frame False {
              }
            }
          }
        }
        n152 = call <vilib>:"Add State(s) to Queue__JKI_lib_State_Machine.vi"("State(s) in (\"\")"=w260) -> ("States Out"=w259:string)  [unwired: 14 in]
      }
      frame "---------- Macro ----------" {
        # "Do not put any code in this frame.\n(It is a separator no-op. You can make a copy of this frame to create a new Macro frame)"
        n153 = call <vilib>:"Add State(s) to Queue__JKI_lib_State_Machine.vi"("State(s) in (\"\")"=w329) -> ("States Out"=w328:string)  [unwired: 14 in]
      }
      frame "Macro: Initialize" {
        w330 = "Data: Initialize\nInitialize Core Data\nUI: Initialize\nUI: Front Panel State >> Open\n\nCFSSL: Find EXE\nCFSSL: Load Certification Authority\nCFSSL: Read CA Certificates\nCFSSL: Validate CA Certificates\nCFSSL: Create Temp Folder\nUI: List Certificates\nUI: Display Selected Certificate\nUI: Refresh"  # Data: Initialize Initialize Core Data UI: Initialize UI: Front Panel State >> Open  CFSSL: Find EXE CFSSL: Load Certification Authority CFSSL: Read CA Certificates CFSSL: Validate CA Certificates CFSSL: Create Temp Folder UI: List Certificates UI: Display Selected Certificate UI: Refresh
        # "Initialization Macro\n(This is called once, when the VI starts)"
        n154 = call <vilib>:"Add State(s) to Queue__JKI_lib_State_Machine.vi"("State(s) in Front (\"\")"=w330, "State(s) in (\"\")"=w334) -> ("States Out"=w333:string)  [unwired: 13 in]
      }
      frame "Macro: Generate Certification Authority" {
        n155 = call <vilib>:"Add State(s) to Queue__JKI_lib_State_Machine.vi"("State(s) in Front (\"\")"="CFSSL: Create Temp Folder\nCFSSL: Prepare CA Request File\nCFSSL: Generate Certification Authority\nCFSSL: Save CA Certificate\nCFSSL: Load Certification Authority\nCFSSL: Read CA Certificates\nCFSSL: Validate CA Certificates\nUI: Refresh\nUI: List Certificates\nUI: Display Selected Certificate", "State(s) in (\"\")"=w339) -> ("States Out"=w338:string)  [unwired: 13 in]
      }
      frame "Macro: Generate Server Certificate" {
        n156 = Bundle By Name(cluster=w343, "Processing Queue"="Servers") -> (w342:T11)
        n157 = call <vilib>:"Add State(s) to Queue__JKI_lib_State_Machine.vi"("State(s) in Front (\"\")"="CFSSL: Create Temp Folder\nCFSSL: Prepare Gencert Config File\nCFSSL: Copy Temporary CA Certificate\n\nMacro: Process Next Server", "State(s) in (\"\")"=w347, "State(s) at Back (\"\")"="UI: Refresh\nUI: List Certificates\nUI: Display Selected Certificate") -> ("States Out"=w346:string)  [unwired: 12 in]
      }
      frame "Macro: Export Root Bundle" {
        n158 = call <vilib>:"Add State(s) to Queue__JKI_lib_State_Machine.vi"("State(s) in Front (\"\")"="CFSSL: Export Root Certificate\nCFSSL: Export Root Private Key\nCFSSL: Export Root Signing Request", "State(s) in (\"\")"=w352) -> ("States Out"=w351:string)  [unwired: 13 in]
      }
      frame "Macro: Process Next Server" {
        n159 = Unbundle By Name(w358) -> ("Processing Queue"=w357:cluster{"hosts":string[], "name":string}[])
        n160 = Empty Array?(array=w357) -> (empty?=w356:bool)
        n161 = Select(t="UI: Refresh", s=w356, f="CFSSL: Load Next Server\nCFSSL: Prepare Server Request File\nCFSSL: Generate Server Certificate\nCFSSL: Save Temporary Server Certificate\nMacro: Process Next Server") -> (s? t:f=w353:string)
        n162 = call <vilib>:"Add State(s) to Queue__JKI_lib_State_Machine.vi"("State(s) in Front (\"\")"=w353, "State(s) in (\"\")"=w361) -> ("States Out"=w360:string)  [unwired: 13 in]
      }
      frame "Macro: Export Server Bundle" {
        n163 = call <vilib>:"Add State(s) to Queue__JKI_lib_State_Machine.vi"("State(s) in Front (\"\")"="CFSSL: Export Server Certificate\nCFSSL: Export Server Private Key\nCFSSL: Export Server Signing Request", "State(s) in (\"\")"=w366) -> ("States Out"=w365:string)  [unwired: 13 in]
      }
      frame "Macro: Exit" {
        # "Exit Macro\n(This is called once, when the VI exits)"
        n164 = Unbundle By Name(w374) -> ("Core.Close Panel on Exit?"=w373:bool)
        n165 = Select(t="UI: Front Panel State >> Close", s=w373, f="") -> (s? t:f=w370:string)
        n166 = call <vilib>:"Add State(s) to Queue__JKI_lib_State_Machine.vi"("State(s) in Front (\"\")"="CFSSL: Delete Temp Folder", "State(s) in (\"\")"=w370, "State(s) at Back (\"\")"="Data: Cleanup\nExit") -> ("States Out"=w368:string)  [unwired: 12 in]
        n167 = call <vilib>:"Add State(s) to Queue__JKI_lib_State_Machine.vi"("State(s) in Front (\"\")"=w368, "State(s) in (\"\")"=w377) -> ("States Out"=w376:string)  [unwired: 13 in]
      }
      frame "---------- Cloudflare SSL ----------" {
        n168 = call <vilib>:"Add State(s) to Queue__JKI_lib_State_Machine.vi"("State(s) in (\"\")"=w381) -> ("States Out"=w380:string)  [unwired: 14 in]
      }
      frame "CFSSL: Find EXE" {
        # "Linux\nMac\nnull\nPharLap\nVxWorks\nWin"
        n169 = disable-structure shown="OS==Win" {
          disable-tunnel: [w393 _] -> w383
          frame condition #0 (active) {
            n170 = call "LVOS Certificates Folder.vi"() -> ("cfssl path"=w395:path)  [unwired: 10 in, 1 out]
            n171 = call <userlib>:"Create Dir if Non-Existant__ogtk.vi"("Directory Path"=w395) -> ("dup Directory Path"=w396:path)  [unwired: 8 in, 2 out]
            n172 = Build Path(base path=w396, name or relative path=path "cfssl.exe") -> (appended path=w393:path)
          }
          frame condition #1 {
          }
        }
        n173 = call-poly <userlib>:"File Exists__ogtk.vi"("file path"=w383) -> ("is directory"=w387:bool, "exists"=w386:bool)  [unwired: 6 in]
        n174 = Compound Arithmetic op=OR(invert w387, w386) -> (w385:bool)
        n175 = Select(t=w383, s=w385, f=path "") -> (s? t:f=w384:path)
        n176 = Bundle By Name(cluster=w389, "cfssl path"=w384) -> (w388:T11)
        n177 = call <vilib>:"Add State(s) to Queue__JKI_lib_State_Machine.vi"("State(s) in (\"\")"=w392) -> ("States Out"=w391:string)  [unwired: 14 in]
      }
      frame "CFSSL: Create Temp Folder" {
        n178 = call <userlib>:"Temporary Directory__ogtk.vi"("Relative path (.)"=path "LV_CFSSL") -> ("Temporary Directory (+ Relative)"=w400:path)
        n179 = call <userlib>:"Create Dir if Non-Existant__ogtk.vi"("error in (no error)"=w399, "Directory Path"=w400) -> ("error out"=w398:errorcluster, "dup Directory Path"=w397:path)  [unwired: 7 in, 1 out]
        n180 = Bundle By Name(cluster=w403, "temp folder"=w397) -> (w402:T11)
        n181 = call <vilib>:"Add State(s) to Queue__JKI_lib_State_Machine.vi"("State(s) in (\"\")"=w405) -> ("States Out"=w404:string)  [unwired: 14 in]
      }
      frame "CFSSL: Delete Temp Folder" {
        n182 = Unbundle By Name(w413) -> ("temp folder"=w407:path)
        n183 = Empty String/Path?(string/path=w407) -> (empty?=w406:bool)
        n184 = call-poly <userlib>:"File Exists__ogtk.vi"("file path"=w407) -> ("is directory"=w411:bool, "exists"=w412:bool)  [unwired: 6 in]
        n185 = Compound Arithmetic op=AND(w411, w412, invert w406) -> (w410:bool)
        n186 = case shown="True" w410 {
          tunnel: w407 -> [_ w420]
          tunnel: [w416 w418] -> w409
          tunnel: w408 -> [w416 w419]
          frame False {
          }
          frame True {
            w417 = TRUE ("Recursive? (FALSE)")
            n187 = call <userlib>:"Delete Recursive__ogtk.vi"("error in (no error)"=w419, "Ignore Read-Only? (FALSE)"=w417, "Recursive? (FALSE)"=w417, "Path"=w420) -> ("error out"=w418:errorcluster)  [unwired: 6 in, 1 out]
          }
        }
        n188 = call <vilib>:"Add State(s) to Queue__JKI_lib_State_Machine.vi"("State(s) in (\"\")"=w415) -> ("States Out"=w414:string)  [unwired: 14 in]
      }
      frame "CFSSL: Load Certification Authority" {
        n189 = Unbundle By Name(w438) -> ("Certificates Folder"=w422:path)
        n190 = Build Path(base path=w422, name or relative path="root.crt") -> (appended path=w423:path)
        n191 = Build Path(base path=w422, name or relative path="root-key.pem") -> (appended path=w421:path)
        n192 = call-poly <userlib>:"File Exists__ogtk.vi"("file path"=w423) -> ("is directory"=w436:bool, "exists"=w435:bool)  [unwired: 6 in]
        n193 = Empty String/Path?(string/path=w423) -> (empty?=w434:bool)
        n194 = call-poly <userlib>:"File Exists__ogtk.vi"("file path"=w421) -> ("is directory"=w426:bool, "exists"=w427:bool)  [unwired: 6 in]
        n195 = Empty String/Path?(string/path=w421) -> (empty?=w428:bool)
        n196 = Compound Arithmetic op=AND(invert w436, w435, invert w434) -> (w433:bool)
        n197 = Compound Arithmetic op=AND(invert w426, w427, invert w428) -> (w429:bool)
        n198 = Select(t=w423, s=w433, f=path "") -> (s? t:f=w431:path)
        n199 = Select(t=w421, s=w429, f=path "") -> (s? t:f=w424:path)
        n200 = Bundle By Name(cluster=w438, "Root Certificate"=w431, "Root Private Key"=w424) -> (w439:T11)
        n201 = call <vilib>:"Add State(s) to Queue__JKI_lib_State_Machine.vi"("State(s) in (\"\")"=w442) -> ("States Out"=w441:string)  [unwired: 14 in]
      }
      frame "CFSSL: Generate Certification Authority" {
        n202 = Unbundle By Name(w446) -> ("cfssl path"=w452:path, "temp folder"=w451:path)
        n203 = Format Into String(format string="\"%s\" gencert -initca csr-ca.json", w452) -> (resulting string=w454:string)  [unwired: 2 in, 1 out]
        n204 = call <vilib>:"System Exec.vi"("run minimized? (F)"=TRUE, "error in (no error)"=w444, "working directory"=w451, "command line"=w454) -> ("error out"=w449:errorcluster, "standard output"=w450:string)  [unwired: 4 in, 2 out]
        n205 = Unbundle By Name(w446) -> ("CA"=w445:T10)
        n206 = Unflatten From JSON(JSON string=w450, type and defaults=w445, error in (no error)=w449) -> (value=w448:T10, error out=w443:errorcluster)  [unwired: 4 in]
        n207 = Bundle By Name(cluster=w446, "CA"=w448) -> (w447:T11)
        n208 = call <vilib>:"Add State(s) to Queue__JKI_lib_State_Machine.vi"("State(s) in (\"\")"=w457) -> ("States Out"=w456:string)  [unwired: 14 in]
      }
      frame "CFSSL: Generate Server Certificate" {
        n209 = Unbundle By Name(w462) -> ("cfssl path"=w468:path, "temp folder"=w467:path)
        n210 = Format Into String(format string="\"%s\" gencert -ca ca.pem -ca-key ca-key.pem -config config.json csr-server.json" ("command line"), w468) -> (resulting string=w469:string)  [unwired: 2 in, 1 out]
        n211 = call <vilib>:"System Exec.vi"("run minimized? (F)"=TRUE, "error in (no error)"=w460, "working directory"=w467, "command line"=w469) -> ("error out"=w465:errorcluster, "standard output"=w466:string)  [unwired: 4 in, 2 out]
        n212 = Unbundle By Name(w462) -> ("Server"=w461:T10)
        n213 = Unflatten From JSON(JSON string=w466, type and defaults=w461, error in (no error)=w465) -> (value=w464:T10, error out=w459:errorcluster)  [unwired: 4 in]
        n214 = Bundle By Name(cluster=w462, "Server"=w464) -> (w463:T11)
        n215 = call <vilib>:"Add State(s) to Queue__JKI_lib_State_Machine.vi"("State(s) in (\"\")"=w472) -> ("States Out"=w471:string)  [unwired: 14 in]
      }
      frame "CFSSL: Prepare CA Request File" {
        (unwired) "{\n    \"CN\": \"lvtls-ca.example\",\n    \"hosts\": [\"lvtls-ca.example\"],\n    \"key\": {\"algo\": \"ecdsa\", \"size\": 256},\n    \"names\": [],\n    \"ca\": {\"pathlen\": 1, \"expiry\": \"143800h\"}\n}" ("name or relative path")
        # "https://github.com/cloudflare/cfssl/wiki/Creating-a-new-CSR"
        n216 = Unbundle By Name(w493) -> ("temp folder"=w492:path)
        n217 = call-poly <userlib>:"Build Path__ogtk.vi"("name or relative path"="csr-ca.json", "base path"=w492) -> ("appended path"=w481:path)
        n218 = Bundle By Name(cluster=T6 {"CN"="", "hosts"=[], "key"={"algo"="ecdsa", "size"=256}, "ca"={"pathlen"=0, "expiry"=""}} ("CSR"), "CN"="Common Name", "hosts"="Hosts", "key.algo"="ecdsa", "key.size"=u32 256, "ca.pathlen"=u8 1, "ca.expiry"="143800h") -> (w487:T6)
        n219 = Flatten To JSON(anything=w487, error in (no error)=w474) -> (JSON string=w479:string, 11:w475:errorcluster)  [unwired: 1 in]
        n220 = Open/Create/Replace File(file path (use dialog)=w481, error in=w475, operation (0:open)=T5."replace or create") -> (refnum out=w480:refnum<file>, error out=w482:errorcluster)  [unwired: 3 in, 1 out]
        n221 = Write to Text File(file (use dialog)=w480, text=w479, error in=w482) -> (refnum out=w476:refnum<file>, error out=w477:errorcluster)  [unwired: 1 in, 1 out]
        n222 = Close File(refnum=w476, error in=w477) -> (error out=w473:errorcluster)  [unwired: 1 out]
        n223 = call <vilib>:"Add State(s) to Queue__JKI_lib_State_Machine.vi"("State(s) in (\"\")"=w495) -> ("States Out"=w494:string)  [unwired: 14 in]
      }
      frame "CFSSL: Prepare Server Request File" {
        (unwired) "{\n    \"CN\": \"lvtls.example\",\n    \"hosts\": [\"lvtls.example\"],\n    \"key\": {\"algo\": \"ecdsa\", \"size\": 256},\n    \"names\": []\n}" ("name or relative path")
        # "https://github.com/cloudflare/cfssl/wiki/Creating-a-new-CSR"
        n224 = Unbundle By Name(w514) -> ("temp folder"=w513:path, "Active CN"=w497:string, "Active Hosts"=w496:string[])
        n225 = call-poly <userlib>:"Build Path__ogtk.vi"("name or relative path"="csr-server.json", "base path"=w513) -> ("appended path"=w510:path)
        n226 = Bundle By Name(cluster=T9 {"CN"="", "hosts"=[], "key"={"algo"="ecdsa", "size"=256}} ("CSR"), "CN"=w497, "hosts"=w496, "key.algo"="ecdsa", "key.size"=u32 256) -> (w499:T9)
        n227 = Flatten To JSON(anything=w499, error in (no error)=w503) -> (JSON string=w508:string, 11:w504:errorcluster)  [unwired: 1 in]
        n228 = Open/Create/Replace File(file path (use dialog)=w510, error in=w504, operation (0:open)=T5."replace or create") -> (refnum out=w509:refnum<file>, error out=w511:errorcluster)  [unwired: 3 in, 1 out]
        n229 = Write to Text File(file (use dialog)=w509, text=w508, error in=w511) -> (refnum out=w505:refnum<file>, error out=w506:errorcluster)  [unwired: 1 in, 1 out]
        n230 = Close File(refnum=w505, error in=w506) -> (error out=w502:errorcluster)  [unwired: 1 out]
        n231 = call <vilib>:"Add State(s) to Queue__JKI_lib_State_Machine.vi"("State(s) in (\"\")"=w516) -> ("States Out"=w515:string)  [unwired: 14 in]
      }
      frame "CFSSL: Copy Temporary CA Certificate" {
        n232 = Unbundle By Name(w526) -> ("Root Certificate"=w530:path, "temp folder"=w531:path)
        n233 = Unbundle By Name(w526) -> ("Root Private Key"=w523:path, "temp folder"=w521:path)
        n234 = call-poly <userlib>:"Build Path__ogtk.vi"("name or relative path"="ca-key.pem", "base path"=w521) -> ("appended path"=w524:path)
        n235 = call-poly <userlib>:"Build Path__ogtk.vi"("name or relative path"="ca.pem", "base path"=w531) -> ("appended path"=w528:path)
        n236 = call <userlib>:"Copy with Options__ogtk.vi"("error in (no error)"=w520, "Replace Mode (Never)"=enum16{"Never", "Always", "If Newer"}."Always", "target path"=w524, "source path"=w523) -> ("error out"=w517:errorcluster)  [unwired: 6 in, 1 out]
        n237 = call <userlib>:"Copy with Options__ogtk.vi"("error in (no error)"=w520, "Replace Mode (Never)"=enum16{"Never", "Always", "If Newer"}."Always", "target path"=w528, "source path"=w530) -> ("error out"=w518:errorcluster)  [unwired: 6 in, 1 out]
        n238 = Merge Errors(w518, w517) -> (w519:errorcluster)
        n239 = call <vilib>:"Add State(s) to Queue__JKI_lib_State_Machine.vi"("State(s) in (\"\")"=w533) -> ("States Out"=w532:string)  [unwired: 14 in]
      }
      frame "CFSSL: Load Next Server" {
        n240 = Unbundle By Name(w538) -> ("Processing Queue"=w537:cluster{"hosts":string[], "name":string}[])
        n241 = Delete From Array(array=w537) -> (deleted portion=w535:cluster{"hosts":string[], "name":string}, array with subset deleted=w536:cluster{"hosts":string[], "name":string}[])  [unwired: 2 in]
        n242 = Unbundle By Name(w535) -> ("name"=w540:string, "hosts"=w539:string[])
        n243 = Bundle By Name(cluster=w538, "Processing Queue"=w536, "Active CN"=w540, "Active Hosts"=w539) -> (w541:T11)
        n244 = call <vilib>:"Add State(s) to Queue__JKI_lib_State_Machine.vi"("State(s) in (\"\")"=w543) -> ("States Out"=w542:string)  [unwired: 14 in]
      }
      frame "CFSSL: Prepare Gencert Config File" {
        n245 = Unbundle By Name(w555) -> ("temp folder"=w554:path)
        n246 = call-poly <userlib>:"Build Path__ogtk.vi"("name or relative path"="config.json", "base path"=w554) -> ("appended path"=w551:path)
        n247 = Open/Create/Replace File(file path (use dialog)=w551, error in=w544, operation (0:open)=T5."replace or create") -> (refnum out=w550:refnum<file>, error out=w552:errorcluster)  [unwired: 3 in, 1 out]
        n248 = Write to Text File(file (use dialog)=w550, text="{\n  \"signing\": {\n       \"default\": {\n           \"expiry\": \"143800h\", \n           \"usages\": [\"server auth\"]\n        }\n    }\n}" ("name or relative path"), error in=w552) -> (refnum out=w547:refnum<file>, error out=w548:errorcluster)  [unwired: 1 in, 1 out]
        n249 = Close File(refnum=w547, error in=w548) -> (error out=w546:errorcluster)  [unwired: 1 out]
        n250 = call <vilib>:"Add State(s) to Queue__JKI_lib_State_Machine.vi"("State(s) in (\"\")"=w557) -> ("States Out"=w556:string)  [unwired: 14 in]
      }
      frame "CFSSL: Save CA Certificate" {
        w566 = T5."replace or create with confirmation" ("operation (0:open)")
        n251 = Unbundle By Name(w558) -> ("Certificates Folder"=w579:path)
        n252 = Unbundle By Name(w558) -> ("CA.cert"=w578:string)
        n253 = Unbundle By Name(w558) -> ("CA.key"=w567:string)
        n254 = Unbundle By Name(w558) -> ("CA.csr"=w568:string)
        n255 = call-poly <userlib>:"Build Path__ogtk.vi"("name or relative path"="root.csr", "base path"=w579) -> ("appended path"=w573:path)
        n256 = call-poly <userlib>:"Build Path__ogtk.vi"("name or relative path"="root.crt", "base path"=w579) -> ("appended path"=w560:path)
        n257 = call-poly <userlib>:"Build Path__ogtk.vi"("name or relative path"="root-key.pem", "base path"=w579) -> ("appended path"=w559:path)
        n258 = Open/Create/Replace File(file path (use dialog)=w573, operation (0:open)=w566) -> (refnum out=w575:refnum<file>, error out=w574:errorcluster)  [unwired: 4 in, 1 out]
        n259 = Open/Create/Replace File(file path (use dialog)=w559, operation (0:open)=w566) -> (refnum out=w571:refnum<file>, error out=w572:errorcluster)  [unwired: 4 in, 1 out]
        n260 = Open/Create/Replace File(file path (use dialog)=w560, operation (0:open)=w566) -> (refnum out=w584:refnum<file>, error out=w585:errorcluster)  [unwired: 4 in, 1 out]
        n261 = Write to Text File(file (use dialog)=w575, text=w568, error in=w574) -> (refnum out=w577:refnum<file>, error out=w576:errorcluster)  [unwired: 1 in, 1 out]
        n262 = Write to Text File(file (use dialog)=w571, text=w567, error in=w572) -> (refnum out=w569:refnum<file>, error out=w570:errorcluster)  [unwired: 1 in, 1 out]
        n263 = Write to Text File(file (use dialog)=w584, text=w578, error in=w585) -> (refnum out=w582:refnum<file>, error out=w583:errorcluster)  [unwired: 1 in, 1 out]
        n264 = Close File(refnum=w577, error in=w576) -> (error out=w563:errorcluster)  [unwired: 1 out]
        n265 = Close File(refnum=w569, error in=w570) -> (error out=w562:errorcluster)  [unwired: 1 out]
        n266 = Close File(refnum=w582, error in=w583) -> (error out=w564:errorcluster)  [unwired: 1 out]
        n267 = Merge Errors(w565, w564, w563, w562) -> (w561:errorcluster)
        n268 = call <vilib>:"Add State(s) to Queue__JKI_lib_State_Machine.vi"("State(s) in (\"\")"=w588) -> ("States Out"=w587:string)  [unwired: 14 in]
      }
      frame "CFSSL: Read CA Certificates" {
        n269 = Unbundle By Name(w604) -> ("Certificates Folder"=w605:path)
        n270 = call-poly <userlib>:"Build Path__ogtk.vi"("name or relative path"="root-key.pem", "base path"=w605) -> ("appended path"=w590:path)
        n271 = call-poly <userlib>:"Build Path__ogtk.vi"("name or relative path"="root.crt", "base path"=w605) -> ("appended path"=w595:path)
        n272 = call-poly <userlib>:"File Exists__ogtk.vi"("file path"=w595) -> ("is directory"=w598:bool, "exists"=w597:bool)  [unwired: 6 in]
        n273 = Empty String/Path?(string/path=w595) -> (empty?=w596:bool)
        n274 = call-poly <userlib>:"File Exists__ogtk.vi"("file path"=w590) -> ("is directory"=w591:bool, "exists"=w592:bool)  [unwired: 6 in]
        n275 = Empty String/Path?(string/path=w590) -> (empty?=w593:bool)
        n276 = Compound Arithmetic op=AND(invert w598, w597, invert w596) -> (w594:bool)
        n277 = Compound Arithmetic op=AND(invert w591, w592, invert w593) -> (w589:bool)
        n278 = case shown="True" w594 {
          tunnel: w595 -> [_ w628]
          tunnel: [_ w624] -> w602
          tunnel: [_ w621] -> w601
          frame False {
          }
          frame True {
            n279 = Open/Create/Replace File(file path (use dialog)=w628, operation (0:open)=T5."open", access (0:read/write)=enum16{"read/write", "read-only", "write-only"}."read-only") -> (refnum out=w627:refnum<file>, error out=w629:errorcluster)  [unwired: 3 in, 1 out]
            n280 = Read from Text File(file (use dialog)=w627, error in=w629) -> (refnum out=w625:refnum<file>, text=w624:string, error out=w626:errorcluster)  [unwired: 2 in, 1 out]
            n281 = Close File(refnum=w625, error in=w626) -> (error out=w621:errorcluster)  [unwired: 1 out]
          }
        }
        n282 = case shown="True" w589 {
          tunnel: w590 -> [_ w616]
          tunnel: [_ w615] -> w600
          tunnel: [_ w612] -> w599
          frame False {
          }
          frame True {
            n283 = Open/Create/Replace File(file path (use dialog)=w616, operation (0:open)=T5."open", access (0:read/write)=enum16{"read/write", "read-only", "write-only"}."read-only") -> (refnum out=w618:refnum<file>, error out=w617:errorcluster)  [unwired: 3 in, 1 out]
            n284 = Read from Text File(file (use dialog)=w618, error in=w617) -> (refnum out=w620:refnum<file>, text=w612:string, error out=w619:errorcluster)  [unwired: 2 in, 1 out]
            n285 = Close File(refnum=w620, error in=w619) -> (error out=w615:errorcluster)  [unwired: 1 out]
          }
        }
        n286 = Bundle By Name(cluster=w604, "CA.cert"=w602, "CA.key"=w599) -> (w603:T11)
        n287 = Merge Errors(w607, w601, w600) -> (w606:errorcluster)
        n288 = call <vilib>:"Add State(s) to Queue__JKI_lib_State_Machine.vi"("State(s) in (\"\")"=w611) -> ("States Out"=w610:string)  [unwired: 14 in]
      }
      frame "CFSSL: Validate CA Certificates" {
        n289 = Unbundle By Name(w633) -> ("Root Certificate"=w631:path, "Root Private Key"=w630:path)  [unwired: 2 out]
        n290 = Bundle By Name(cluster=w633, "Root Certificate"=w631, "Root Private Key"=w630) -> (w632:T11)
        n291 = Merge Errors(w635) -> (w634:errorcluster)
        n292 = call <vilib>:"Add State(s) to Queue__JKI_lib_State_Machine.vi"("State(s) in (\"\")"=w637) -> ("States Out"=w636:string)  [unwired: 14 in]
      }
      frame "CFSSL: Save Temporary CA Certificate" {
        w638 = T5."replace or create" ("operation (0:open)")
        n293 = Unbundle By Name(w650) -> ("temp folder"=w651:path)
        n294 = Unbundle By Name(w650) -> ("CA.cert"=w649:string)
        n295 = Unbundle By Name(w650) -> ("CA.key"=w643:string)
        n296 = call-poly <userlib>:"Build Path__ogtk.vi"("name or relative path"="root.crt", "base path"=w651) -> ("appended path"=w656:path)
        n297 = call-poly <userlib>:"Build Path__ogtk.vi"("name or relative path"="root-key.pem", "base path"=w651) -> ("appended path"=w644:path)
        n298 = Open/Create/Replace File(file path (use dialog)=w644, operation (0:open)=w638) -> (refnum out=w647:refnum<file>, error out=w648:errorcluster)  [unwired: 4 in, 1 out]
        n299 = Open/Create/Replace File(file path (use dialog)=w656, operation (0:open)=w638) -> (refnum out=w655:refnum<file>, error out=w657:errorcluster)  [unwired: 4 in, 1 out]
        n300 = Write to Text File(file (use dialog)=w647, text=w643, error in=w648) -> (refnum out=w645:refnum<file>, error out=w646:errorcluster)  [unwired: 1 in, 1 out]
        n301 = Write to Text File(file (use dialog)=w655, text=w649, error in=w657) -> (refnum out=w653:refnum<file>, error out=w654:errorcluster)  [unwired: 1 in, 1 out]
        n302 = Close File(refnum=w645, error in=w646) -> (error out=w640:errorcluster)  [unwired: 1 out]
        n303 = Close File(refnum=w653, error in=w654) -> (error out=w641:errorcluster)  [unwired: 1 out]
        n304 = Merge Errors(w642, w641, w640) -> (w639:errorcluster)
        n305 = call <vilib>:"Add State(s) to Queue__JKI_lib_State_Machine.vi"("State(s) in (\"\")"=w660) -> ("States Out"=w659:string)  [unwired: 14 in]
      }
      frame "CFSSL: Save Temporary Server Certificate" {
        w680 = T5."replace or create" ("operation (0:open)")
        n306 = Unbundle By Name(w675) -> ("Certificates Folder"=w671:path, "Active CN"=w667:string)
        n307 = Unbundle By Name(w675) -> ("Certificates Folder"=w670:path, "Active CN"=w674:string, "Server.key"=w669:string)
        n308 = Unbundle By Name(w675) -> ("Server.cert"=w661:string, "CA.cert"=w663:string)
        n309 = Format Into String(format string="%s-key.pem", w674) -> (resulting string=w672:string)  [unwired: 2 in, 1 out]
        n310 = Format Into String(format string="%s.crt", w667) -> (resulting string=w668:string)  [unwired: 2 in, 1 out]
        n311 = call-poly <userlib>:"Build Path__ogtk.vi"("name or relative path"=w668, "base path"=w671) -> ("appended path"=w689:path)
        n312 = call-poly <userlib>:"Build Path__ogtk.vi"("name or relative path"=w672, "base path"=w670) -> ("appended path"=w681:path)
        n313 = Open/Create/Replace File(file path (use dialog)=w681, operation (0:open)=w680) -> (refnum out=w684:refnum<file>, error out=w685:errorcluster)  [unwired: 4 in, 1 out]
        n314 = Open/Create/Replace File(file path (use dialog)=w689, operation (0:open)=w680) -> (refnum out=w688:refnum<file>, error out=w690:errorcluster)  [unwired: 4 in, 1 out]
        n315 = Write to Text File(file (use dialog)=w684, text=w669, error in=w685) -> (refnum out=w682:refnum<file>, error out=w683:errorcluster)  [unwired: 1 in, 1 out]
        n316 = Format Into String(format string="%s%s%s", w661, "\n", w663) -> (resulting string=w662:string)  [unwired: 2 in, 1 out]
        n317 = Close File(refnum=w682, error in=w683) -> (error out=w677:errorcluster)  [unwired: 1 out]
        n318 = Write to Text File(file (use dialog)=w688, text=w662, error in=w690) -> (refnum out=w686:refnum<file>, error out=w687:errorcluster)  [unwired: 1 in, 1 out]
        n319 = Close File(refnum=w686, error in=w687) -> (error out=w678:errorcluster)  [unwired: 1 out]
        n320 = Merge Errors(w679, w678, w677) -> (w676:errorcluster)
        n321 = call <vilib>:"Add State(s) to Queue__JKI_lib_State_Machine.vi"("State(s) in (\"\")"=w692) -> ("States Out"=w691:string)  [unwired: 14 in]
      }
      frame "CFSSL: Export Root Private Key" {
        n322 = Unbundle By Name(w701) -> ("Certificates Folder"=w702:path, "Root name"=w695:string)
        n323 = Unbundle By Name(w701) -> ("CA.key"=w700:string)
        n324 = call-poly <userlib>:"Convert File Extension__ogtk.vi"("new ending (none)"="pem" ("format string"), "file name"=w695) -> ("new filename"=w693:string)  [unwired: 1 out]
        n325 = call-poly <userlib>:"Build Path__ogtk.vi"("name or relative path"=w693, "base path"=w702) -> ("appended path"=w706:path)
        n326 = Open/Create/Replace File(file path (use dialog)=w706, operation (0:open)=T5."replace or create with confirmation") -> (refnum out=w705:refnum<file>, error out=w707:errorcluster)  [unwired: 4 in, 1 out]
        n327 = Write to Text File(file (use dialog)=w705, text=w700, error in=w707) -> (refnum out=w703:refnum<file>, error out=w704:errorcluster)  [unwired: 1 in, 1 out]
        n328 = Close File(refnum=w703, error in=w704) -> (error out=w697:errorcluster)  [unwired: 1 out]
        n329 = Merge Errors(w698, w697) -> (w696:errorcluster)
        n330 = call <vilib>:"Add State(s) to Queue__JKI_lib_State_Machine.vi"("State(s) in (\"\")"=w709) -> ("States Out"=w708:string)  [unwired: 14 in]
      }
      frame "CFSSL: Export Root Certificate" {
        n331 = Unbundle By Name(w718) -> ("Certificates Folder"=w719:path, "Root name"=w712:string)
        n332 = Unbundle By Name(w718) -> ("CA.cert"=w717:string)
        n333 = call-poly <userlib>:"Convert File Extension__ogtk.vi"("new ending (none)"="crt" ("format string"), "file name"=w712) -> ("new filename"=w710:string)  [unwired: 1 out]
        n334 = call-poly <userlib>:"Build Path__ogtk.vi"("name or relative path"=w710, "base path"=w719) -> ("appended path"=w723:path)
        n335 = Open/Create/Replace File(file path (use dialog)=w723, operation (0:open)=T5."replace or create with confirmation") -> (refnum out=w722:refnum<file>, error out=w724:errorcluster)  [unwired: 4 in, 1 out]
        n336 = Write to Text File(file (use dialog)=w722, text=w717, error in=w724) -> (refnum out=w720:refnum<file>, error out=w721:errorcluster)  [unwired: 1 in, 1 out]
        n337 = Close File(refnum=w720, error in=w721) -> (error out=w714:errorcluster)  [unwired: 1 out]
        n338 = Merge Errors(w715, w714) -> (w713:errorcluster)
        n339 = call <vilib>:"Add State(s) to Queue__JKI_lib_State_Machine.vi"("State(s) in (\"\")"=w726) -> ("States Out"=w725:string)  [unwired: 14 in]
      }
      frame "CFSSL: Export Root Signing Request" {
        n340 = Unbundle By Name(w735) -> ("Certificates Folder"=w736:path, "Root name"=w729:string)
        n341 = Unbundle By Name(w735) -> ("CA.csr"=w734:string)
        n342 = call-poly <userlib>:"Convert File Extension__ogtk.vi"("new ending (none)"="csr" ("format string"), "file name"=w729) -> ("new filename"=w727:string)  [unwired: 1 out]
        n343 = call-poly <userlib>:"Build Path__ogtk.vi"("name or relative path"=w727, "base path"=w736) -> ("appended path"=w740:path)
        n344 = Open/Create/Replace File(file path (use dialog)=w740, operation (0:open)=T5."replace or create with confirmation") -> (refnum out=w739:refnum<file>, error out=w741:errorcluster)  [unwired: 4 in, 1 out]
        n345 = Write to Text File(file (use dialog)=w739, text=w734, error in=w741) -> (refnum out=w737:refnum<file>, error out=w738:errorcluster)  [unwired: 1 in, 1 out]
        n346 = Close File(refnum=w737, error in=w738) -> (error out=w731:errorcluster)  [unwired: 1 out]
        n347 = Merge Errors(w732, w731) -> (w730:errorcluster)
        n348 = call <vilib>:"Add State(s) to Queue__JKI_lib_State_Machine.vi"("State(s) in (\"\")"=w743) -> ("States Out"=w742:string)  [unwired: 14 in]
      }
      frame "CFSSL: Export Server Certificate" {
        n349 = Unbundle By Name(w752) -> ("Certificates Folder"=w753:path, "Root name"=w746:string)
        n350 = Unbundle By Name(w752) -> ("Server.cert"=w751:string)
        n351 = call-poly <userlib>:"Convert File Extension__ogtk.vi"("new ending (none)"="cer" ("format string"), "file name"=w746) -> ("new filename"=w744:string)  [unwired: 1 out]
        n352 = call-poly <userlib>:"Build Path__ogtk.vi"("name or relative path"=w744, "base path"=w753) -> ("appended path"=w757:path)
        n353 = Open/Create/Replace File(file path (use dialog)=w757, operation (0:open)=T5."replace or create with confirmation") -> (refnum out=w756:refnum<file>, error out=w758:errorcluster)  [unwired: 4 in, 1 out]
        n354 = Write to Text File(file (use dialog)=w756, text=w751, error in=w758) -> (refnum out=w754:refnum<file>, error out=w755:errorcluster)  [unwired: 1 in, 1 out]
        n355 = Close File(refnum=w754, error in=w755) -> (error out=w748:errorcluster)  [unwired: 1 out]
        n356 = Merge Errors(w749, w748) -> (w747:errorcluster)
        n357 = call <vilib>:"Add State(s) to Queue__JKI_lib_State_Machine.vi"("State(s) in (\"\")"=w760) -> ("States Out"=w759:string)  [unwired: 14 in]
      }
      frame "CFSSL: Export Server Private Key" {
        n358 = Unbundle By Name(w769) -> ("Certificates Folder"=w770:path, "Root name"=w763:string)
        n359 = Unbundle By Name(w769) -> ("Server.key"=w768:string)
        n360 = call-poly <userlib>:"Convert File Extension__ogtk.vi"("new ending (none)"="pem" ("format string"), "file name"=w763) -> ("new filename"=w761:string)  [unwired: 1 out]
        n361 = call-poly <userlib>:"Build Path__ogtk.vi"("name or relative path"=w761, "base path"=w770) -> ("appended path"=w774:path)
        n362 = Open/Create/Replace File(file path (use dialog)=w774, operation (0:open)=T5."replace or create with confirmation") -> (refnum out=w773:refnum<file>, error out=w775:errorcluster)  [unwired: 4 in, 1 out]
        n363 = Write to Text File(file (use dialog)=w773, text=w768, error in=w775) -> (refnum out=w771:refnum<file>, error out=w772:errorcluster)  [unwired: 1 in, 1 out]
        n364 = Close File(refnum=w771, error in=w772) -> (error out=w765:errorcluster)  [unwired: 1 out]
        n365 = Merge Errors(w766, w765) -> (w764:errorcluster)
        n366 = call <vilib>:"Add State(s) to Queue__JKI_lib_State_Machine.vi"("State(s) in (\"\")"=w777) -> ("States Out"=w776:string)  [unwired: 14 in]
      }
      frame "CFSSL: Export Server Signing Request" {
        n367 = Unbundle By Name(w786) -> ("Certificates Folder"=w787:path, "Root name"=w780:string)
        n368 = Unbundle By Name(w786) -> ("Server.csr"=w785:string)
        n369 = call-poly <userlib>:"Convert File Extension__ogtk.vi"("new ending (none)"="csr" ("format string"), "file name"=w780) -> ("new filename"=w778:string)  [unwired: 1 out]
        n370 = call-poly <userlib>:"Build Path__ogtk.vi"("name or relative path"=w778, "base path"=w787) -> ("appended path"=w791:path)
        n371 = Open/Create/Replace File(file path (use dialog)=w791, operation (0:open)=T5."replace or create with confirmation") -> (refnum out=w790:refnum<file>, error out=w792:errorcluster)  [unwired: 4 in, 1 out]
        n372 = Write to Text File(file (use dialog)=w790, text=w785, error in=w792) -> (refnum out=w788:refnum<file>, error out=w789:errorcluster)  [unwired: 1 in, 1 out]
        n373 = Close File(refnum=w788, error in=w789) -> (error out=w782:errorcluster)  [unwired: 1 out]
        n374 = Merge Errors(w783, w782) -> (w781:errorcluster)
        n375 = call <vilib>:"Add State(s) to Queue__JKI_lib_State_Machine.vi"("State(s) in (\"\")"=w794) -> ("States Out"=w793:string)  [unwired: 14 in]
      }
    }
  }
